vi "Main5states.vi"() -> ()   [LabVIEW 2021]
uses:
  controls/SynchroCheckCentral.ctl
  controls/SynchroCheckCentral_Info.ctl
  controls/SynchroCheckCentral_Data.ctl
  controls/3ph Phasor.ctl
  controls/Phasor.ctl
  controls/AFE_froming_Central.ctl
  controls/AFE_froming_Central_Info.ctl
  controls/AFE_froming_Central_Data.ctl
  controls/references.ctl
  controls/Connected_OPF.ctl
  controls/Connected_OPF_Info.ctl
  controls/Connected_OPF_Data.ctl
  controls/PVemulator_Central.ctl
  controls/PVemulator_Central_Info.ctl
  controls/PVemulator_Central_Data.ctl
  controls/measurements.ctl
  controls/measurements_SC.ctl
  controls/SC_references.ctl
  controls/MeteoBoxCentral.ctl
  controls/MeteoBoxCentral_Info.ctl
  controls/MeteoBoxCentral_Data.ctl
  controls/Setpoints_CDA.ctl
  controls/Setpoints_CDA_ZENONE.ctl
  controls/SCADA_to_SM.ctl
  controls/SCADAOGCentral_Info.ctl
  controls/SCADA_to_SM_Data.ctl
  controls/State Machine.ctl
  <vilib>/Platform/TimedLoop/XDataNode/timing_clust.ctl
  <vilib>/Platform/TimedLoop/XDataNode/nitl_modes.ctl
  <vilib>/Platform/TimedLoop/XDataNode/wakeup.ctl
  controls/PV_facade_central.ctl
  controls/PV_facade_cental_Info.ctl
  controls/PV_facade_central_Data.ctl
  controls/state_2.ctl
  <vilib>/Analysis/baseanly.llb/Mean (DBL).vi
  <vilib>/JDP Science/JSONtext/Next JSON Value.vi
  <vilib>/JDP Science/JSONtext/String Subset.vi
  <vilib>/JDP Science/JSONtext/Parsing/Advance past next JSON Value (inlined COPY).vi
  <vilib>/JDP Science/JSONtext/Parsing/Advance past whitespace.vi
  <vilib>/JDP Science/JSONtext/Parsing/Advance past String.vi
  <vilib>/JDP Science/JSONtext/Parsing/Advance past Number.vi
  <vilib>/JDP Science/JSONtext/Parsing/Advance past Line Ending.vi
  <vilib>/JDP Science/JSONtext/Parsing/Parse Full Path or Item Name.vi
  <vilib>/JDP Science/JSONtext/Parsing/Advance past Array.vi
  <vilib>/JDP Science/JSONtext/Parsing/Advance past Object.vi
  <vilib>/JDP Science/JSONtext/support/Error Cluster From Code.vi
  <vilib>/JDP Science/JSONtext/Offset/Find Item Locations by Path.vi
  <vilib>/Utility/file.llb/Read Delimited Spreadsheet (DBL).vi
  <vilib>/Platform/TimedLoop/TimeConversion.llb/rt-milliseconds-to-rel-time.vi
  <vilib>/Platform/TimedLoop/XDataNode/XDataNode.xnode
  <vilib>/Platform/TimedLoop/XDataNode/XDNodeRunTimeDep.lvlib
  <vilib>/JDP Science/JSONtext/JSONtext.lvlib
  <userlib>/_OpenG.lib/boolean/boolean.llb/openg_boolean__ogtk.lvlib
  <vilib>/ptbypt/NI_PtbyPt.lvlib
  <vilib>/Analysis/NI_AALBase.lvlib
panel:
  in  "IN cOPF 2":T1={"Info"={"Resource"="Zenone", "Problem"=0.0, "Timestamp"=0.0}, "Data"={"Operation_mode"="Grid connected", "solution_feasible"=0.0, "Optimal_slack"="AFE 1", "setpoints"=[], "upper_layer_grid_info"={"Frequency"=0.0, "Angle"=0.0, "Magnitude"=0.0}, "SC_soc"=0.0, "PV"={"perun"=0.0, "solarmax"=0.0, "facade"=0.0, "emul4"=0.0, "emul5"=0.0, "emul6"=0.0, "emul7"=0.0}, "P_pv_facade"=0.0}}
  out "OUT cOPF 2":T1={"Info"={"Resource"="Zenone", "Problem"=0.0, "Timestamp"=0.0}, "Data"={"Operation_mode"="Grid connected", "solution_feasible"=0.0, "Optimal_slack"="AFE 1", "setpoints"=[], "upper_layer_grid_info"={"Frequency"=0.0, "Angle"=0.0, "Magnitude"=0.0}, "SC_soc"=0.0, "PV"={"perun"=0.0, "solarmax"=0.0, "facade"=0.0, "emul4"=0.0, "emul5"=0.0, "emul6"=0.0, "emul7"=0.0}, "P_pv_facade"=0.0}}
  in  "Stop 2":bool
  out "Iteration Duration":dbl
  out "old_sp_island_bool":bool=TRUE
  out "old_sp_island":dbl[](array[numeric])
  out "V_freq_for_island":dbl
  out "V_freq":dbl
  out "V angle":cluster{"output":dbl}(graph)
  in  "Reset_angle":bool
  in  "SampleSize 2":u8=33
  out "SOC":cluster{"mean":dbl}(graph)
  out "V_control_fix_for_island":dbl
  out "V control":cluster{"output":dbl}(graph)
  out "V_control":dbl
  out "V_afe":dbl
  out "V_upstream":dbl
  in  "Reset_magnitude":bool
  out "SCADA data":bool
  in  "SCADA":T4={"Info"={"Resource"="MeteoBox", "Problem"=FALSE, "Timestamp"=0.0}, "Data"={"Voltage mag"=[], "Voltage angle"=[]}}
  in  "to connected-island":bool
  in  "OUT":T7
  in  "Real_SOC":bool
  out "time connected":timestamp
  out "time island":timestamp
  out "P_bess_island":dbl
  out "P_bess_connected":dbl
  out "P_pv_facade":dbl
  in  "SOC":dbl=40.0
  in  "IN Meteo":T9={"Info"={"Resource"="MeteoBox", "Problem"=FALSE, "Timestamp"=0.0}, "Data"={"GI"=0.0, "GHI"=0.0, "GVI"=0.0, "Tair"=0.0, "Tcell roof"=0.0, "Global_Total_Irr"=0.0, "Diffused_Irr"=0.0, "Tcell facade"=0.0, "PV_mpp"={"perun"=0.0, "solarmax"=0.0, "facade"=0.0, "emul4"=0.0, "emul5"=0.0, "emul6"=0.0, "emul7"=0.0}}}
  out "SC_soc":dbl
  out "delta angle":dbl
  in  "Send sp DC?":bool
  in  "Send sp AC?":bool
  out "Zenone_Q":dbl
  out "Zenone_P":dbl
  out "forming SC?":bool
  out "OUT PV+SC":T12={"Info"={"Resource"="Zenone", "Problem"=FALSE, "Timestamp"=0.0}, "Data"={"Status 1"=FALSE, "Status 2"=FALSE, "measurements"={"V_PV1"=0.0, "V_CAP1"=0.0, "V_PV2"=0.0, "V_CAP2"=0.0, "V_grid2"=0.0, "V_PV3"=0.0, "V_CAP3"=0.0, "V_grid3"=0.0, "V_PV4"=0.0, "V_CAP4"=0.0, "V_grid4"=0.0, "V_grid1"=0.0, "P1"=0.0, "P2"=0.0, "P3"=0.0, "P4"=0.0}, "Status 3"=FALSE, "Status 4"=FALSE, "measurements SC"={"V_SC"=0.0, "V_CAP"=0.0, "V_grid"=0.0, "P"=0.0, "SOC"=0.0}, "Status SC"=FALSE, "Forming/Following"=FALSE, "Start forming"=FALSE, "SC references"={"Vdc"=0.0, "Pdc"=0.0}, "Start following"=FALSE}}
  out "PV data":bool
  out "AFE data":bool
  out "synchro data":bool
  in  "IN PV+SC":T12={"Info"={"Resource"="Zenone", "Problem"=FALSE, "Timestamp"=0.0}, "Data"={"Status 1"=FALSE, "Status 2"=FALSE, "measurements"={"V_PV1"=0.0, "V_CAP1"=0.0, "V_PV2"=0.0, "V_CAP2"=0.0, "V_grid2"=0.0, "V_PV3"=0.0, "V_CAP3"=0.0, "V_grid3"=0.0, "V_PV4"=0.0, "V_CAP4"=0.0, "V_grid4"=0.0, "V_grid1"=0.0, "P1"=0.0, "P2"=0.0, "P3"=0.0, "P4"=0.0}, "Status 3"=FALSE, "Status 4"=FALSE, "measurements SC"={"V_SC"=0.0, "V_CAP"=0.0, "V_grid"=0.0, "P"=0.0, "SOC"=0.0}, "Status SC"=FALSE, "Forming/Following"=FALSE, "Start forming"=FALSE, "SC references"={"Vdc"=0.0, "Pdc"=0.0}, "Start following"=FALSE}}
  out "iOPF data":bool
  out "cOPF data":bool
  in  "IN AFE":T18={"Info"={"Resource"="Zenone", "Problem"=FALSE, "Timestamp"=0.0}, "Data"={"Start forming 1"=FALSE, "Forming/Following"=[], "Start forming 2"=FALSE, "measurements"={"Vdc1"=0.0, "P1"=0.0, "Vdc2"=0.0, "P2"=0.0, "Q2"=0.0, "Vdc3"=0.0, "P3"=0.0, "Q3"=0.0, "Vdc4"=0.0, "P4"=0.0, "Q4"=0.0, "Q1"=0.0}, "Status"=[], "references"={"Vdc1"=0.0, "Vdc2"=0.0, "Qac2"=0.0, "Vdc3"=0.0, "Qac3"=0.0, "Vdc4"=0.0, "Qac4"=0.0, "Qac1"=0.0, "V_arg2"=0.0, "V_abs2"=0.0, "V_abs1"=0.0, "V_arg1"=0.0, "freq1"=0.0, "freq2"=0.0}, "Start following 1"=FALSE, "Start following 2"=FALSE}}
  in  "IN cOPF":T1={"Info"={"Resource"="Zenone", "Problem"=0.0, "Timestamp"=0.0}, "Data"={"Operation_mode"="Grid connected", "solution_feasible"=0.0, "Optimal_slack"="AFE 1", "setpoints"=[], "upper_layer_grid_info"={"Frequency"=0.0, "Angle"=0.0, "Magnitude"=0.0}, "SC_soc"=0.0, "PV"={"perun"=0.0, "solarmax"=0.0, "facade"=0.0, "emul4"=0.0, "emul5"=0.0, "emul6"=0.0, "emul7"=0.0}, "P_pv_facade"=0.0}}
  in  "IN iOPF":T1={"Info"={"Resource"="Zenone", "Problem"=0.0, "Timestamp"=0.0}, "Data"={"Operation_mode"="Grid connected", "solution_feasible"=0.0, "Optimal_slack"="AFE 1", "setpoints"=[], "upper_layer_grid_info"={"Frequency"=0.0, "Angle"=0.0, "Magnitude"=0.0}, "SC_soc"=0.0, "PV"={"perun"=0.0, "solarmax"=0.0, "facade"=0.0, "emul4"=0.0, "emul5"=0.0, "emul6"=0.0, "emul7"=0.0}, "P_pv_facade"=0.0}}
  in  "IN synchro":T22={"Info"={"Resource"="SyncroCheck", "Problem"=FALSE, "Timestamp"=0.0}, "Data"={"close/open relay"=TRUE, "Operation mode"="Grid connected", "V_Downstream"={"Phase A"={"Frequency"=0.0, "Magnitude"=0.0, "Angle [Deg]"=0.0}, "Phase B"={"Frequency"=0.0, "Magnitude"=0.0, "Angle [Deg]"=0.0}, "Phase C"={"Frequency"=0.0, "Magnitude"=0.0, "Angle [Deg]"=0.0}, "Phase N"={"Frequency"=0.0, "Magnitude"=0.0, "Angle [Deg]"=0.0}}, "V_UpStream"={"Phase A"={"Frequency"=0.0, "Magnitude"=0.0, "Angle [Deg]"=0.0}, "Phase B"={"Frequency"=0.0, "Magnitude"=0.0, "Angle [Deg]"=0.0}, "Phase C"={"Frequency"=0.0, "Magnitude"=0.0, "Angle [Deg]"=0.0}, "Phase N"={"Frequency"=0.0, "Magnitude"=0.0, "Angle [Deg]"=0.0}}, "Synchronised?"=TRUE}}
  out "OUT iOPF":T1={"Info"={"Resource"="Zenone", "Problem"=0.0, "Timestamp"=0.0}, "Data"={"Operation_mode"="Grid connected", "solution_feasible"=0.0, "Optimal_slack"="AFE 1", "setpoints"=[], "upper_layer_grid_info"={"Frequency"=0.0, "Angle"=0.0, "Magnitude"=0.0}, "SC_soc"=0.0, "PV"={"perun"=0.0, "solarmax"=0.0, "facade"=0.0, "emul4"=0.0, "emul5"=0.0, "emul6"=0.0, "emul7"=0.0}, "P_pv_facade"=0.0}}
  out "OUT cOPF":T1={"Info"={"Resource"="Zenone", "Problem"=0.0, "Timestamp"=0.0}, "Data"={"Operation_mode"="Grid connected", "solution_feasible"=0.0, "Optimal_slack"="AFE 1", "setpoints"=[], "upper_layer_grid_info"={"Frequency"=0.0, "Angle"=0.0, "Magnitude"=0.0}, "SC_soc"=0.0, "PV"={"perun"=0.0, "solarmax"=0.0, "facade"=0.0, "emul4"=0.0, "emul5"=0.0, "emul6"=0.0, "emul7"=0.0}, "P_pv_facade"=0.0}}
  out "OUT AFE":T18={"Info"={"Resource"="Zenone", "Problem"=FALSE, "Timestamp"=0.0}, "Data"={"Start forming 1"=FALSE, "Forming/Following"=[], "Start forming 2"=FALSE, "measurements"={"Vdc1"=0.0, "P1"=0.0, "Vdc2"=0.0, "P2"=0.0, "Q2"=0.0, "Vdc3"=0.0, "P3"=0.0, "Q3"=0.0, "Vdc4"=0.0, "P4"=0.0, "Q4"=0.0, "Q1"=0.0}, "Status"=[], "references"={"Vdc1"=0.0, "Vdc2"=0.0, "Qac2"=0.0, "Vdc3"=0.0, "Qac3"=0.0, "Vdc4"=0.0, "Qac4"=0.0, "Qac1"=0.0, "V_arg2"=0.0, "V_abs2"=0.0, "V_abs1"=0.0, "V_arg1"=0.0, "freq1"=0.0, "freq2"=0.0}, "Start following 1"=FALSE, "Start following 2"=FALSE}}
  out "OUT Synchro":T22={"Info"={"Resource"="SyncroCheck", "Problem"=FALSE, "Timestamp"=0.0}, "Data"={"close/open relay"=TRUE, "Operation mode"="Grid connected", "V_Downstream"={"Phase A"={"Frequency"=0.0, "Magnitude"=0.0, "Angle [Deg]"=0.0}, "Phase B"={"Frequency"=0.0, "Magnitude"=0.0, "Angle [Deg]"=0.0}, "Phase C"={"Frequency"=0.0, "Magnitude"=0.0, "Angle [Deg]"=0.0}, "Phase N"={"Frequency"=0.0, "Magnitude"=0.0, "Angle [Deg]"=0.0}}, "V_UpStream"={"Phase A"={"Frequency"=0.0, "Magnitude"=0.0, "Angle [Deg]"=0.0}, "Phase B"={"Frequency"=0.0, "Magnitude"=0.0, "Angle [Deg]"=0.0}, "Phase C"={"Frequency"=0.0, "Magnitude"=0.0, "Angle [Deg]"=0.0}, "Phase N"={"Frequency"=0.0, "Magnitude"=0.0, "Angle [Deg]"=0.0}}, "Synchronised?"=TRUE}}
  out "setpoints":dbl[](array[numeric])
  in  "nb instances":i16=7
  out "optimal_slack":string(combo)="AFE 1"
  out "iOPF valid":bool
  out "forming AFE?":bool
  out "cOPF valid?":bool
  out "synchronised?":bool
  in  "to grid connection":bool
  in  "to prepare for grid connection":bool
  in  "to island":bool
  in  "Stop":bool
  in  "to prepare for island":bool
  # "32.58"
  # "Islanding Manoeuvre - State Machine"
  # "synchronised"
  # "opf connected OK"
  # "opf island OK"
  # "forming AFE?"
  # "forming SC?"
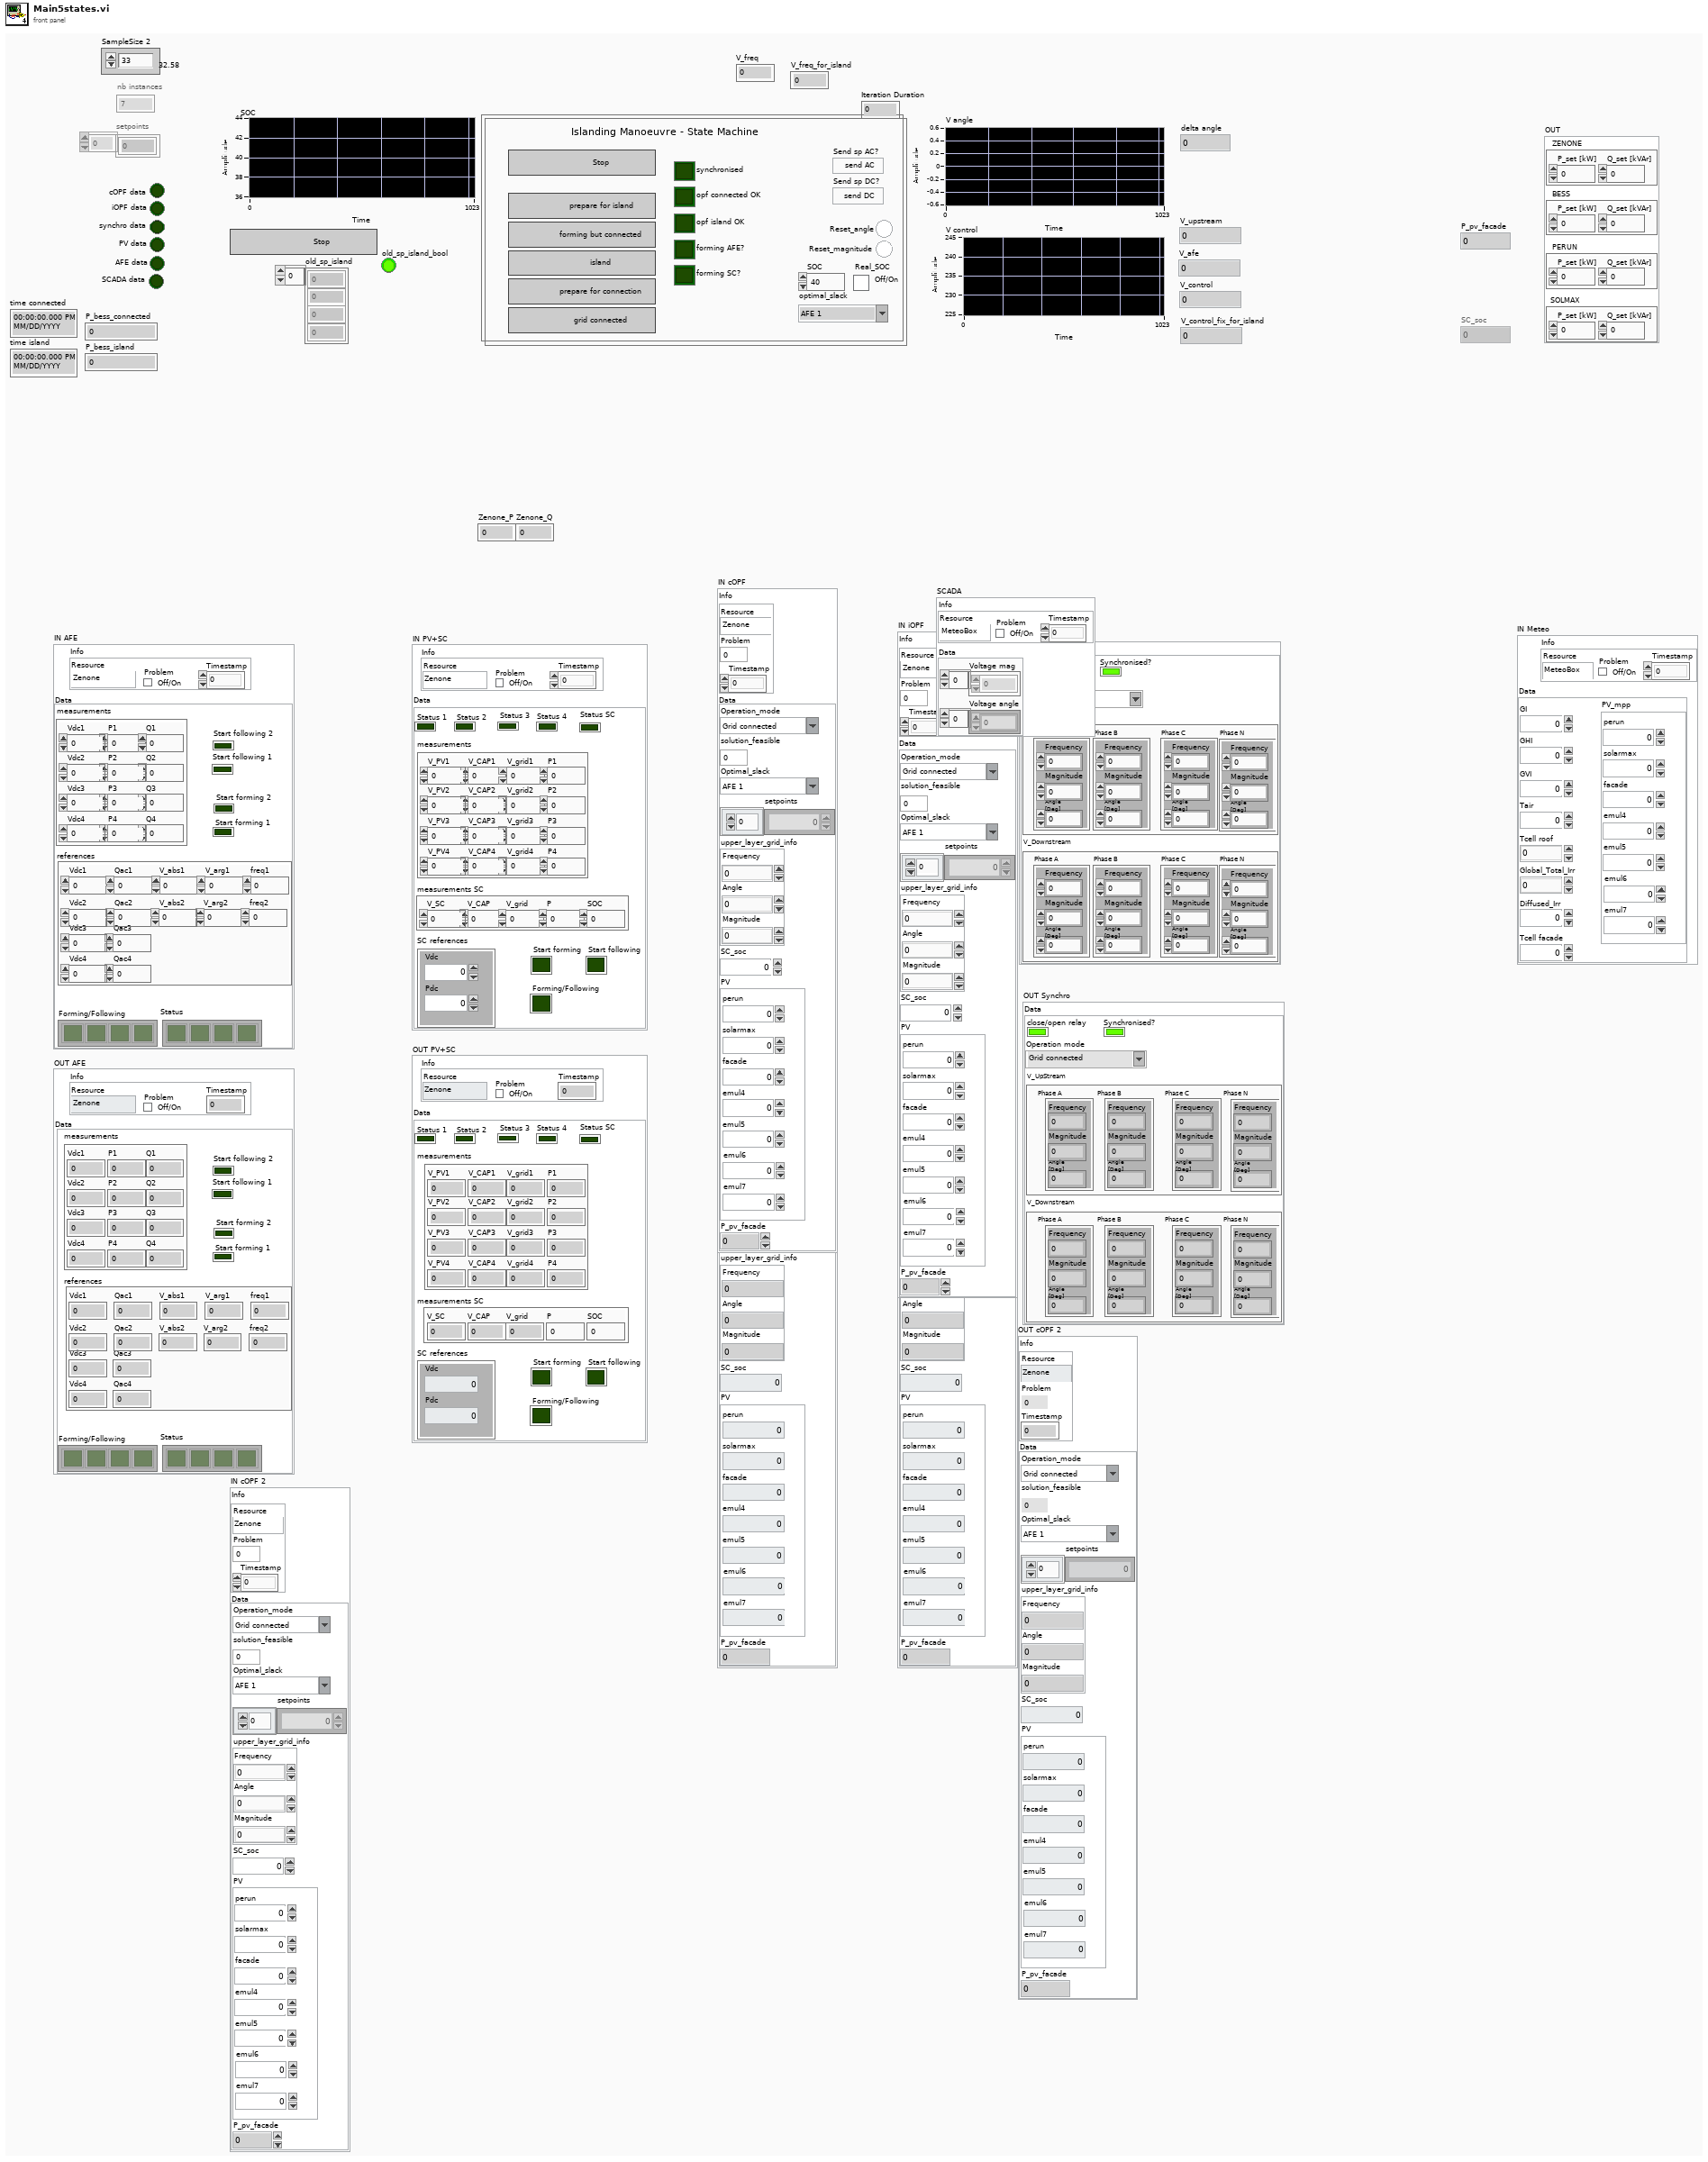
[diagram p1: front panel]
types:
  T1 = typedef "Connected_OPF.ctl" = cluster{"Info":T2, "Data":T3}
  T2 = typedef "Connected_OPF_Info.ctl" = cluster{"Resource":string, "Problem":dbl, "Timestamp":dbl}
  T3 = typedef "Connected_OPF_Data.ctl" = cluster{"Operation_mode":string, "solution_feasible":dbl, "Optimal_slack":string, "setpoints":dbl[], "upper_layer_grid_info":cluster{"Frequency":dbl, "Angle":dbl, "Magnitude":dbl}, "SC_soc":dbl, "PV":cluster{"perun":dbl, "solarmax":dbl, "facade":dbl, "emul4":dbl, "emul5":dbl, "emul6":dbl, "emul7":dbl}, "P_pv_facade":dbl}
  T4 = typedef "SCADA_to_SM.ctl" = cluster{"Info":T5, "Data":T6}
  T5 = typedef "SCADAOGCentral_Info.ctl" = cluster{"Resource":string, "Problem":bool, "Timestamp":dbl}
  T6 = typedef "SCADA_to_SM_Data.ctl" = cluster{"Voltage mag":dbl[], "Voltage angle":dbl[]}
  T7 = typedef "Setpoints_CDA.ctl" = cluster{"ZENONE":T8, "BESS":T8, "PERUN":T8, "SOLMAX":T8}
  T8 = typedef "Setpoints_CDA_ZENONE.ctl" = cluster{"P_set [kW]":dbl, "Q_set [kVAr]":dbl}
  T9 = typedef "MeteoBoxCentral.ctl" = cluster{"Info":T10, "Data":T11}
  T10 = typedef "MeteoBoxCentral_Info.ctl" = cluster{"Resource":string, "Problem":bool, "Timestamp":dbl}
  T11 = typedef "MeteoBoxCentral_Data.ctl" = cluster{"GI":dbl, "GHI":dbl, "GVI":dbl, "Tair":dbl, "Tcell roof":dbl, "Global_Total_Irr":dbl, "Diffused_Irr":dbl, "Tcell facade":dbl, "PV_mpp":cluster{"perun":dbl, "solarmax":dbl, "facade":dbl, "emul4":dbl, "emul5":dbl, "emul6":dbl, "emul7":dbl}}
  T12 = typedef "PVemulator_Central.ctl" = cluster{"Info":T13, "Data":T14}
  T13 = typedef "PVemulator_Central_Info.ctl" = cluster{"Resource":string, "Problem":bool, "Timestamp":dbl}
  T14 = typedef "PVemulator_Central_Data.ctl" = cluster{"Status 1":bool, "Status 2":bool, "measurements":T15, "Status 3":bool, "Status 4":bool, "measurements SC":T16, "Status SC":bool, "Forming/Following":bool, "Start forming":bool, "SC references":T17, "Start following":bool}
  T15 = typedef "measurements.ctl" = cluster{"V_PV1":dbl, "V_CAP1":dbl, "V_PV2":dbl, "V_CAP2":dbl, "V_grid2":dbl, "V_PV3":dbl, "V_CAP3":dbl, "V_grid3":dbl, "V_PV4":dbl, "V_CAP4":dbl, "V_grid4":dbl, "V_grid1":dbl, "P1":dbl, "P2":dbl, "P3":dbl, "P4":dbl}
  T16 = typedef "measurements_SC.ctl" = cluster{"V_SC":dbl, "V_CAP":dbl, "V_grid":dbl, "P":dbl, "SOC":dbl}
  T17 = typedef "SC_references.ctl" = cluster{"Vdc":dbl, "Pdc":dbl}
  T18 = typedef "AFE_froming_Central.ctl" = cluster{"Info":T19, "Data":T20}
  T19 = typedef "AFE_froming_Central_Info.ctl" = cluster{"Resource":string, "Problem":bool, "Timestamp":dbl}
  T20 = typedef "AFE_froming_Central_Data.ctl" = cluster{"Start forming 1":bool, "Forming/Following":bool[], "Start forming 2":bool, "measurements":cluster{"Vdc1":dbl, "P1":dbl, "Vdc2":dbl, "P2":dbl, "Q2":dbl, "Vdc3":dbl, "P3":dbl, "Q3":dbl, "Vdc4":dbl, "P4":dbl, "Q4":dbl, "Q1":dbl}, "Status":bool[], "references":T21, "Start following 1":bool, "Start following 2":bool}
  T21 = typedef "references.ctl" = cluster{"Vdc1":dbl, "Vdc2":dbl, "Qac2":dbl, "Vdc3":dbl, "Qac3":dbl, "Vdc4":dbl, "Qac4":dbl, "Qac1":dbl, "V_arg2":dbl, "V_abs2":dbl, "V_abs1":dbl, "V_arg1":dbl, "freq1":dbl, "freq2":dbl}
  T22 = typedef "SynchroCheckCentral.ctl" = cluster{"Info":T23, "Data":T24}
  T23 = typedef "SynchroCheckCentral_Info.ctl" = cluster{"Resource":string, "Problem":bool, "Timestamp":dbl}
  T24 = typedef "SynchroCheckCentral_Data.ctl" = cluster{"close/open relay":bool, "Operation mode":string, "V_Downstream":T25, "V_UpStream":T25, "Synchronised?":bool}
  T25 = typedef "3ph Phasor.ctl" = cluster{"Phase A":T26, "Phase B":T26, "Phase C":T26, "Phase N":T26}
  T26 = typedef "Phasor.ctl" = cluster{"Frequency":dbl, "Magnitude":dbl, "Angle [Deg]":dbl}
  T27 = typedef "State Machine.ctl" = enum16{"Grid connected", "Prepare for island", "Forming but connected", "Island", "Prepare for connection"}
  T28 = typedef "XDNodeRunTimeDep.lvlib/timing_clust.ctl" = cluster{"Expected End [f-1]":u64, "Actual End [f-1]":u64, "Finished Late? [f-1]":bool, "Expected End [i-1]":u64, "Actual End [i-1]":u64, "Finished Late? [i-1]":bool, "Expected Start [i]":u64, "Actual Start [i]":u64, "Expected Start [f]":u64, "Actual Start [f]":u64, "Source Name":string, "Structure Name":string, "Period":i64, "Deadline":i64, "Offset":i64, "Start":i64, "Priority":i32, "Timeout":i32, "Mode":T29, "Wakeup Reason":T30, "Error":errorcluster, "Source Type":string, "Secondary Source Type":string, "Global End Time":u64, "Global Start Time":u64, "Frame Duration":u64, "Iteration Duration":u64, "Assigned CPU":i32, "I/O Scan Engine Mode":u32}
  T29 = typedef "XDNodeRunTimeDep.lvlib/nitl_modes.ctl" = enum32{"No Change", "Process missed periods, maintain original phase", "Discard missed periods, maintain original phase", "Process missed periods, ignore original phase", "Discard missed periods, ignore original phase"}
  T30 = typedef "XDNodeRunTimeDep.lvlib/wakeup.ctl" = enum32{"Normal", "Aborted", "Asynchronous wakeup", "Timing source error", "Timed loop error", "Timeout"}
  T31 = typedef "PV_facade_central.ctl" = cluster{"Info":T32, "Data":T33}
  T32 = typedef "PV_facade_cental_Info.ctl" = cluster{"Resource":string, "Problem":bool, "Timestamp":dbl}
  T33 = typedef "PV_facade_central_Data.ctl" = cluster{"P":dbl, "Q":dbl, "Pset":dbl, "Qset":dbl}
  T34 = typedef "state_2.ctl" = string
  T35 = cluster{"Frequency":dbl, "Angle":dbl, "Magnitude":dbl}
  T36 = cluster{"perun":dbl, "solarmax":dbl, "facade":dbl, "emul4":dbl, "emul5":dbl, "emul6":dbl, "emul7":dbl}
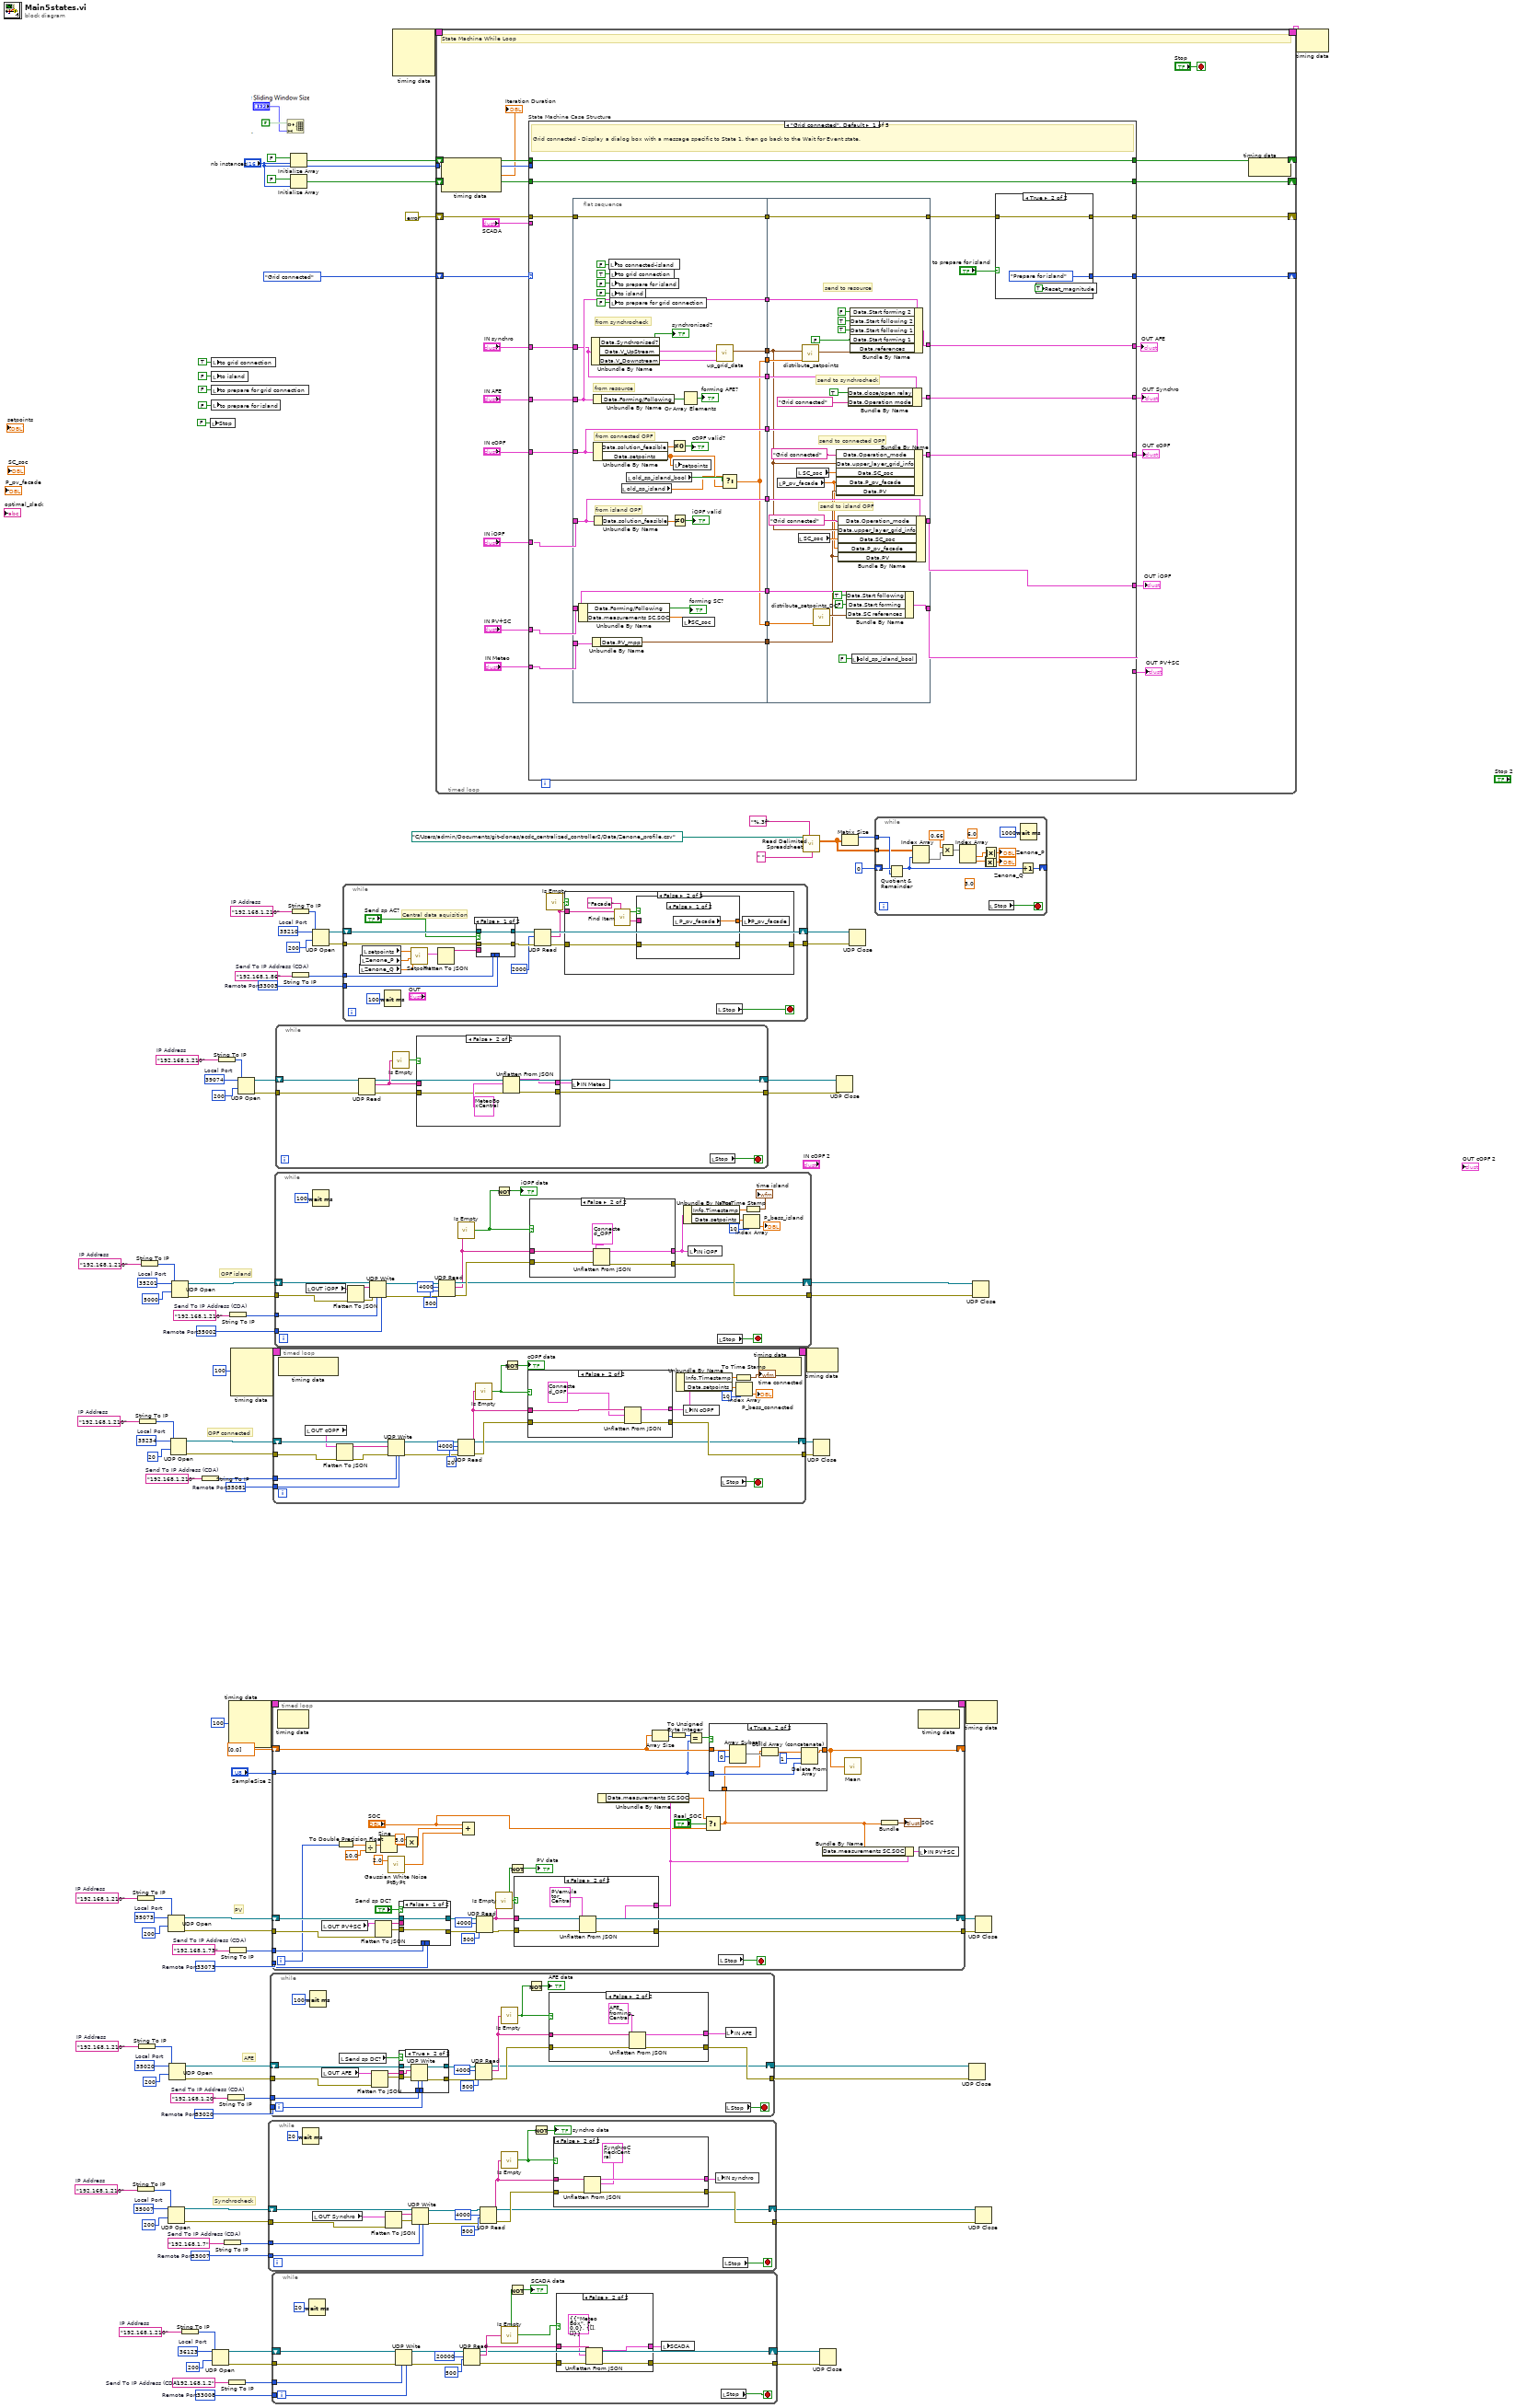
[diagram p0: block diagram]
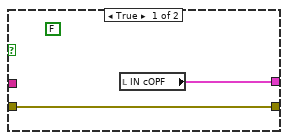
[diagram p2: hidden frame]
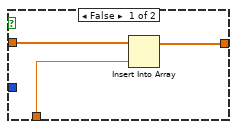
[diagram p3: hidden frame]
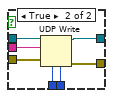
[diagram p4: hidden frame]
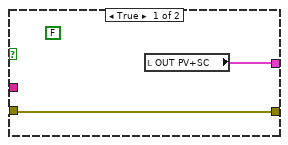
[diagram p5: hidden frame]
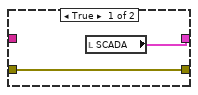
[diagram p6: hidden frame]
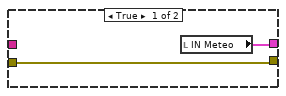
[diagram p7: hidden frame]
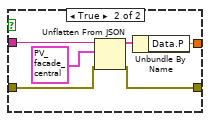
[diagram p9: hidden frame]
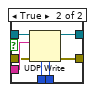
[diagram p10: hidden frame]
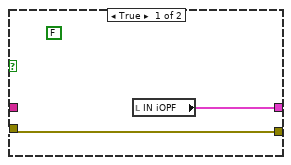
[diagram p11: hidden frame]
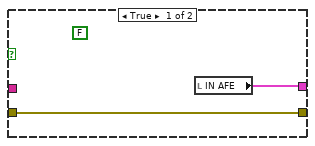
[diagram p13: hidden frame]
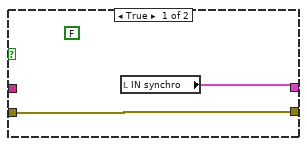
[diagram p14: hidden frame]
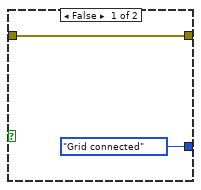
[diagram p15: hidden frame]
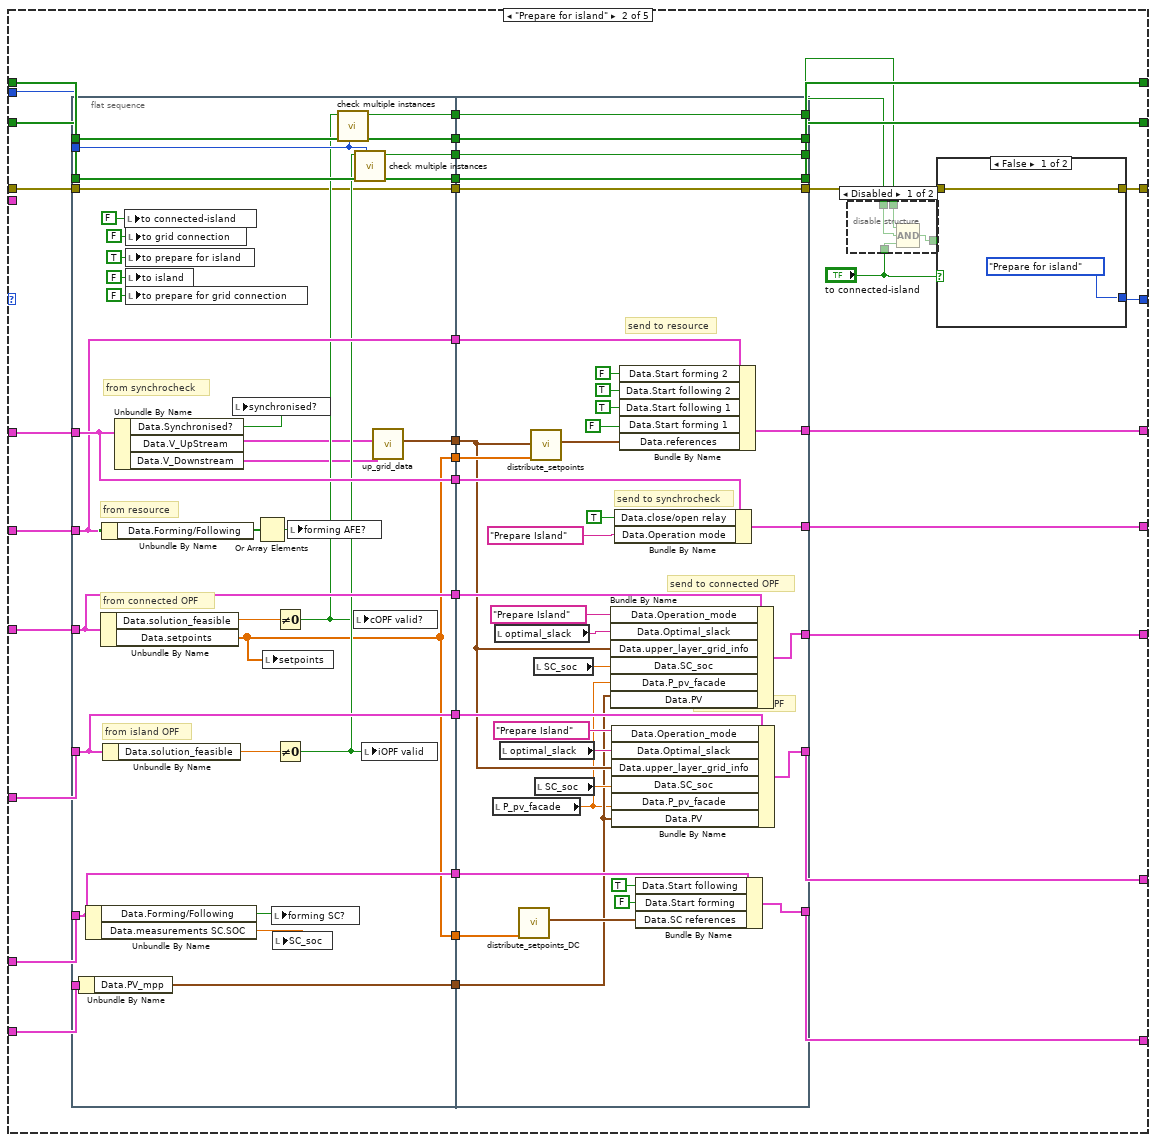
[diagram p16: hidden frame]
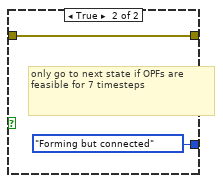
[diagram p18: hidden frame]
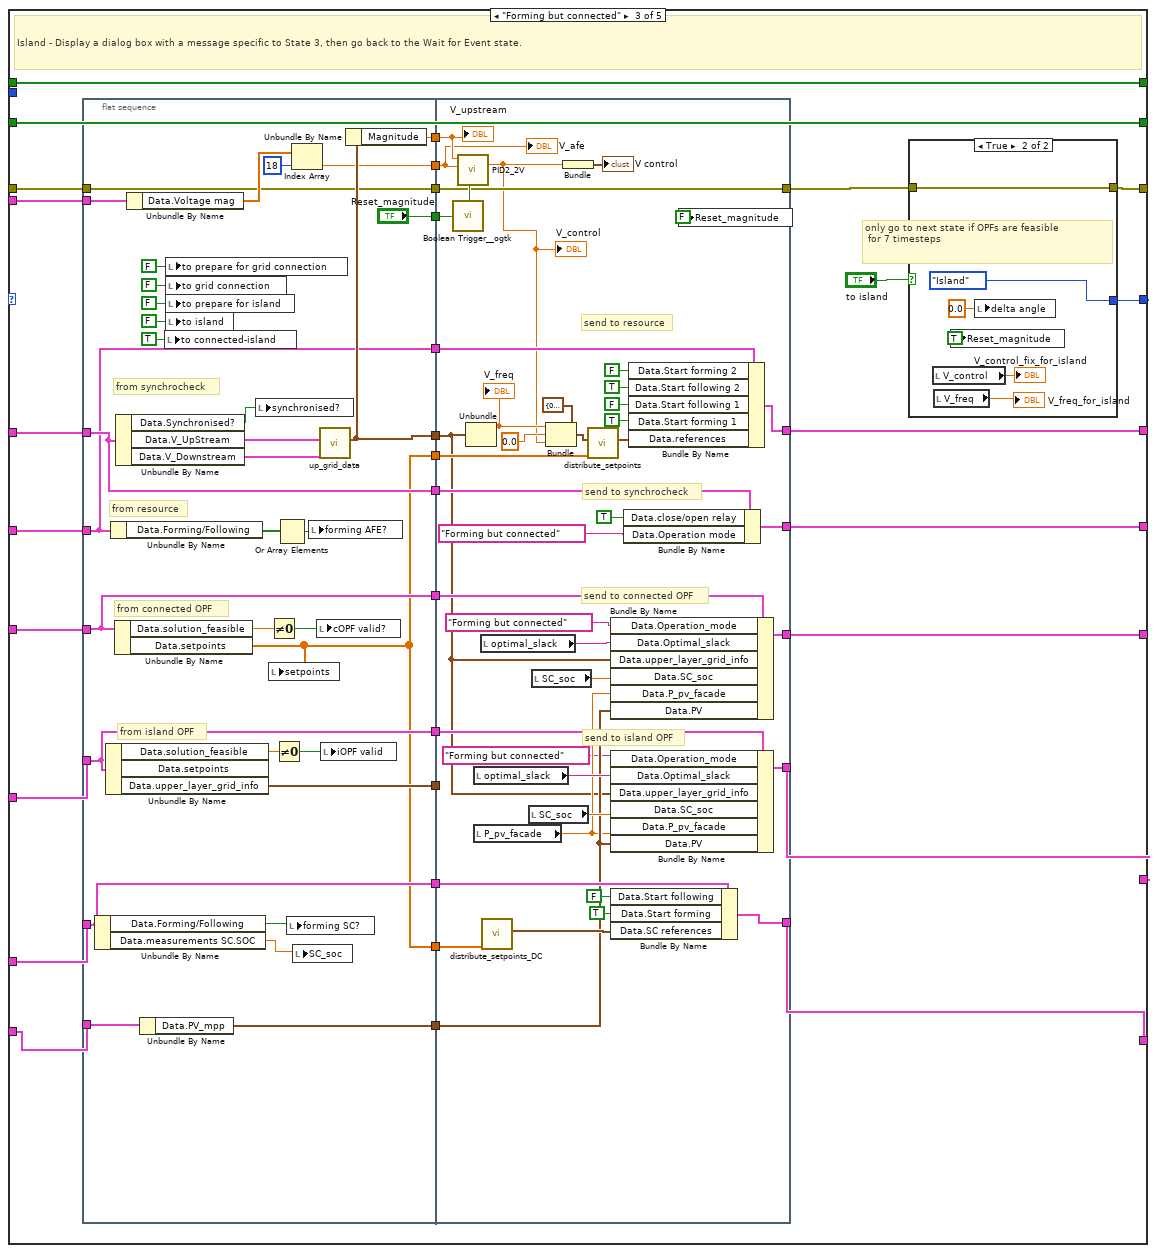
[diagram p19: hidden frame]
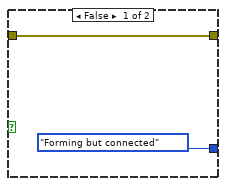
[diagram p20: hidden frame]
diagram:
  w1 = u16 35081  # Remote Port
  w3 = "192.168.1.210"  # Send To IP Address (CDA)
  w15 = u16 33008  # Remote Port
  w19 = "192.168.1.2"  # Send To IP Address (CDA)
  w20 = u16 36123  # Local Port
  w22 = "192.168.1.210"  # IP Address
  w29 = u16 39074  # Local Port
  w31 = "192.168.1.210"  # IP Address
  w40 = u16 33003  # Remote Port
  w42 = "192.168.1.86"  # Send To IP Address (CDA)
  w44 = u16 35210  # Local Port
  w46 = "192.168.1.210"  # IP Address
  w68 = u16 33073  # Remote Port
  w69 = "192.168.1.73"  # Send To IP Address (CDA)
  w64 = u16 33020  # Remote Port
  w72 = "192.168.1.20"  # Send To IP Address (CDA)
  w59 = u16 33007  # Remote Port
  w73 = "192.168.1.7"  # Send To IP Address (CDA)
  w74 = u16 35007  # Local Port
  w76 = "192.168.1.210"  # IP Address
  w78 = u16 35020  # Local Port
  w80 = "192.168.1.210"  # IP Address
  w82 = u16 35073  # Local Port
  w84 = "192.168.1.210"  # IP Address
  w87 = u16 35002  # Remote Port
  w88 = "192.168.1.210"  # Send To IP Address (CDA)
  w95 = u16 35234  # Local Port
  w97 = "192.168.1.210"  # IP Address
  w101 = u16 35201  # Local Port
  w103 = "192.168.1.210"  # IP Address
  # "Synchrocheck"
  # "AFE"
  # "PV"
  # "OPF connected"
  # "OPF island"
  n1 = String To IP(1:w76) -> (0:w77:u32)
  n2 = String To IP(1:w84) -> (0:w85:u32)
  n3 = String To IP(1:w80) -> (0:w81:u32)
  n4 = String To IP(1:w97) -> (0:w98:u32)
  n5 = String To IP(1:w103) -> (0:w104:u32)
  n6 = UDP Open(7:w77, 9:200 ("timeout ms (25000)"), 11:w74) -> (port=w62:refnum<k16>, 0:w61:errorcluster)  [unwired: 2 in, 1 out]
  n7 = UDP Open(7:w85, 9:200 ("timeout ms (25000)"), 11:w82) -> (port=w71:refnum<k16>, 0:w70:errorcluster)  [unwired: 2 in, 1 out]
  n8 = UDP Open(7:w81, 9:200 ("timeout ms (25000)"), 11:w78) -> (port=w66:refnum<k16>, 0:w65:errorcluster)  [unwired: 2 in, 1 out]
  n9 = UDP Open(7:w98, 9:20 ("timeout ms (25000)"), 11:w95) -> (port=w94:refnum<k16>, 0:w93:errorcluster)  [unwired: 2 in, 1 out]
  n10 = UDP Open(7:w104, 9:5000 ("timeout ms (25000)"), 11:w101) -> (port=w100:refnum<k16>, 0:w99:errorcluster)  [unwired: 2 in, 1 out]
  n11 = String To IP(1:w22) -> (0:w23:u32)
  n12 = String To IP(1:w3) -> (0:w2:u32)
  n13 = local write "Stop"(FALSE ("Stop")) -> ()
  n14 = local write "to grid connection"(TRUE ("to grid connection")) -> ()
  n15 = local write "to island"(FALSE ("to island")) -> ()
  n16 = local write "to prepare for grid connection"(FALSE ("to prepare for grid connection")) -> ()
  n17 = local write "to prepare for island"(FALSE ("to prepare for island")) -> ()
  n18 = UDP Open(7:w23, 9:200 ("timeout ms (25000)"), 11:w20) -> (port=w18:refnum<k16>, 0:w17:errorcluster)  [unwired: 2 in, 1 out]
  n19 = String To IP(1:w31) -> (0:w32:u32)
  n20 = String To IP(1:w73) -> (0:w60:u32)
  n21 = String To IP(1:w72) -> (0:w63:u32)
  n22 = node-c288(i64 100 ("Period")) -> (w9:T28)  [unwired: 3 in]
  n23 = String To IP(1:w19) -> (0:w16:u32)
  n24 = String To IP(1:w69) -> (0:w67:u32)
  n25 = String To IP(1:w88) -> (0:w86:u32)
  n26 = node-c288(i64 100 ("Period")) -> (w6:T28)  [unwired: 3 in]
  n27 = UDP Open(7:w32, 9:200 ("timeout ms (25000)"), 11:w29) -> (port=w28:refnum<k16>, 0:w27:errorcluster)  [unwired: 2 in, 1 out]
  n28 = while {
    tunnel: w60 -> [w133]
    tunnel: w59 -> [w132]
    shift-right: [w118] -> w58
    shift-left: w62 -> [w116]
    tunnel: w61 -> [w114]
    tunnel: [w119] -> w57
    stop <- w121 stop-if-true
    n29 = Wait (ms)(milliseconds to wait=u32 20) -> ()  [unwired: 1 out]
    n30 = local read "OUT Synchro"() -> (w126:T22)
    n31 = Flatten To JSON(anything=w126, error in (no error)=w114) -> (JSON string=w120:string, 11:w127:errorcluster)  [unwired: 1 in]
    n32 = UDP Write(address=w133, port or service name=w132, connection ID=w116, data in=w120, 8:w127) -> (error out=w115:errorcluster, 3:w117:refnum<k16>)  [unwired: 1 in]
    n33 = UDP Read(connection ID=w117, max size (548)=4000, timeout ms (25000)=500, 8:w115) -> (data out=w131:string, error out=w123:errorcluster, 3:w118:refnum<k16>)  [unwired: 2 out]
    n34 = call <vilib>:"Is Empty.vi"("JSON"=w131) -> ("Empty"=w124:bool)  [unwired: 4 in]
    n35 = Not(x=w124) -> (.not. x?=→"synchro data":bool)
    n36 = case shown="False" w124 {
      tunnel: w123 -> [w135 w137]
      tunnel: [w134 w140] -> w128
      tunnel: w131 -> [_ w136]
      tunnel: [w135 w139] -> w119
      frame True {
        (unwired) FALSE ("Found")
        n37 = local read "IN synchro"() -> (w134:T22)
      }
      frame False {
        n38 = Unflatten From JSON(JSON string=w136, type and defaults=T22 {"Info"={"Resource"="SyncroCheck", "Problem"=FALSE, "Timestamp"=0.0}, "Data"={"close/open relay"=TRUE, "Operation mode"="Grid connected", "V_Downstream"={"Phase A"={"Frequency"=0.0, "Magnitude"=0.0, "Angle [Deg]"=0.0}, "Phase B"={"Frequency"=0.0, "Magnitude"=0.0, "Angle [Deg]"=0.0}, "Phase C"={"Frequency"=0.0, "Magnitude"=0.0, "Angle [Deg]"=0.0}, "Phase N"={"Frequency"=0.0, "Magnitude"=0.0, "Angle [Deg]"=0.0}}, "V_UpStream"={"Phase A"={"Frequency"=0.0, "Magnitude"=0.0, "Angle [Deg]"=0.0}, "Phase B"={"Frequency"=0.0, "Magnitude"=0.0, "Angle [Deg]"=0.0}, "Phase C"={"Frequency"=0.0, "Magnitude"=0.0, "Angle [Deg]"=0.0}, "Phase N"={"Frequency"=0.0, "Magnitude"=0.0, "Angle [Deg]"=0.0}}, "Synchronised?"=TRUE}} ("IN synchro"), error in (no error)=w137) -> (value=w140:T22, error out=w139:errorcluster)  [unwired: 4 in]
      }
    }
    n39 = local write "IN synchro"(w128) -> ()
    n40 = local read "Stop"() -> (w121:bool)
  }
  n41 = while {
    tunnel: w64 -> [w161]
    tunnel: w63 -> [w160]
    shift-right: [w144] -> w54
    shift-left: w66 -> [w146]
    tunnel: w65 -> [w148]
    tunnel: [w150] -> w53
    stop <- w152 stop-if-true
    n42 = Wait (ms)(milliseconds to wait=u32 100) -> ()  [unwired: 1 out]
    n43 = local read "OUT AFE"() -> (w143:T18)
    n44 = local read "Send sp DC?"() -> (w141:bool)
    n45 = Flatten To JSON(anything=w143, error in (no error)=w148) -> (JSON string=w151:string, 11:w156:errorcluster)  [unwired: 1 in]
    n46 = case shown="True" w141 {
      tunnel: w161 -> [_ w170]
      tunnel: w160 -> [_ w169]
      tunnel: w156 -> [w162 w168]
      tunnel: w151 -> [_ w167]
      tunnel: [w162 w166] -> w149
      tunnel: [w163 w165] -> w147
      tunnel: w146 -> [w163 w164]
      frame False {
      }
      frame True {
        n47 = UDP Write(address=w169, port or service name=w170, connection ID=w164, data in=w167, 8:w168) -> (error out=w166:errorcluster, 3:w165:refnum<k16>)  [unwired: 1 in]
      }
    }
    n48 = UDP Read(connection ID=w147, max size (548)=4000, timeout ms (25000)=500, 8:w149) -> (data out=w145:string, error out=w157:errorcluster, 3:w144:refnum<k16>)  [unwired: 2 out]
    n49 = call <vilib>:"Is Empty.vi"("JSON"=w145) -> ("Empty"=w154:bool)  [unwired: 4 in]
    n50 = Not(x=w154) -> (.not. x?=→"AFE data":bool)
    n51 = case shown="False" w154 {
      tunnel: w157 -> [w172 w176]
      tunnel: [w171 w174] -> w142
      tunnel: w145 -> [_ w175]
      tunnel: [w172 w177] -> w150
      frame True {
        (unwired) FALSE ("Found")
        n52 = local read "IN AFE"() -> (w171:T18)
      }
      frame False {
        n53 = Unflatten From JSON(JSON string=w175, type and defaults=T18 {"Info"={"Resource"="Zenone", "Problem"=FALSE, "Timestamp"=0.0}, "Data"={"Start forming 1"=FALSE, "Forming/Following"=[], "Start forming 2"=FALSE, "measurements"={"Vdc1"=0.0, "P1"=0.0, "Vdc2"=0.0, "P2"=0.0, "Q2"=0.0, "Vdc3"=0.0, "P3"=0.0, "Q3"=0.0, "Vdc4"=0.0, "P4"=0.0, "Q4"=0.0, "Q1"=0.0}, "Status"=[], "references"={"Vdc1"=0.0, "Vdc2"=0.0, "Qac2"=0.0, "Vdc3"=0.0, "Qac3"=0.0, "Vdc4"=0.0, "Qac4"=0.0, "Qac1"=0.0, "V_arg2"=0.0, "V_abs2"=0.0, "V_abs1"=0.0, "V_arg1"=0.0, "freq1"=0.0, "freq2"=0.0}, "Start following 1"=FALSE, "Start following 2"=FALSE}} ("IN AFE"), error in (no error)=w176) -> (value=w174:T18, error out=w177:errorcluster)  [unwired: 4 in]
      }
    }
    n54 = local write "IN AFE"(w142) -> ()
    n55 = local read "Stop"() -> (w152:bool)
  }
  n56 = timed-loop {
    tunnel: w68 -> [w218]
    tunnel: w67 -> [w201]
    shift-right: [w206] -> w56
    shift-left: w71 -> [w209]
    tunnel: w70 -> [w205]
    tunnel: [w203] -> w55
    shift-right: [w185] -> _
    shift-left: dbl[] [0.0] -> [w187]
    tunnel: "SampleSize 2" -> [w179]
    timing: w9 -> [_]
    timing-out: [_] -> w8
    i -> [w186]
    stop <- w210 stop-if-true
    n57 = node-c288() -> ()  [unwired: 1 in, 1 out]
    n58 = local read "OUT PV+SC"() -> (w202:T12)
    n59 = To Double Precision Float(number=w186) -> (double precision float=w198:dbl)
    n60 = Divide(x=w198, y=10.0) -> (x/y=w197:dbl)
    n61 = Flatten To JSON(anything=w202, error in (no error)=w205) -> (JSON string=w211:string, 11:w214:errorcluster)  [unwired: 1 in]
    n62 = Sine(x=w197) -> (sin(x)=w195:dbl)
    n63 = call <vilib>:"Gaussian White Noise PtByPt.vi"("standard deviation"=2.0) -> ("Gaussian white noise"=w194:dbl)  [unwired: 2 in]
    n64 = case shown="False" "Send sp DC?" {
      tunnel: w218 -> [_ w240]
      tunnel: w201 -> [_ w239]
      tunnel: w214 -> [w232 w238]
      tunnel: w211 -> [_ w237]
      tunnel: w209 -> [w233 w236]
      tunnel: [w233 w235] -> w207
      tunnel: [w232 w234] -> w204
      frame False {
      }
      frame True {
        n65 = UDP Write(address=w239, port or service name=w240, connection ID=w236, data in=w237, 8:w238) -> (error out=w234:errorcluster, 3:w235:refnum<k16>)  [unwired: 1 in]
      }
    }
    n66 = Multiply(x=5.0, y=w195) -> (x*y=w192:dbl)
    n67 = Compound Arithmetic op=ADD("SOC", w192, w194) -> ()  [unwired: 1 out]
    n68 = UDP Read(connection ID=w207, max size (548)=4000, timeout ms (25000)=500, 8:w204) -> (data out=w217:string, error out=w215:errorcluster, 3:w206:refnum<k16>)  [unwired: 2 out]
    n69 = call <vilib>:"Is Empty.vi"("JSON"=w217) -> ("Empty"=w212:bool)  [unwired: 4 in]
    n70 = Not(x=w212) -> (.not. x?=→"PV data":bool)
    n71 = case shown="False" w212 {
      tunnel: w215 -> [w242 w245]
      tunnel: [w241 w247] -> w182
      tunnel: w217 -> [_ w244]
      tunnel: [w242 w246] -> w203
      frame True {
        (unwired) FALSE ("Found")
        n72 = local read "OUT PV+SC"() -> (w241:T12)
      }
      frame False {
        n73 = Unflatten From JSON(JSON string=w244, type and defaults=T12 {"Info"={"Resource"="Zenone", "Problem"=FALSE, "Timestamp"=0.0}, "Data"={"Status 1"=FALSE, "Status 2"=FALSE, "measurements"={"V_PV1"=0.0, "V_CAP1"=0.0, "V_PV2"=0.0, "V_CAP2"=0.0, "V_grid2"=0.0, "V_PV3"=0.0, "V_CAP3"=0.0, "V_grid3"=0.0, "V_PV4"=0.0, "V_CAP4"=0.0, "V_grid4"=0.0, "V_grid1"=0.0, "P1"=0.0, "P2"=0.0, "P3"=0.0, "P4"=0.0}, "Status 3"=FALSE, "Status 4"=FALSE, "measurements SC"={"V_SC"=0.0, "V_CAP"=0.0, "V_grid"=0.0, "P"=0.0, "SOC"=0.0}, "Status SC"=FALSE, "Forming/Following"=FALSE, "Start forming"=FALSE, "SC references"={"Vdc"=0.0, "Pdc"=0.0}, "Start following"=FALSE}} ("PV+SC"), error in (no error)=w245) -> (value=w247:T12, error out=w246:errorcluster)  [unwired: 4 in]
      }
    }
    n74 = Unbundle By Name(w182) -> ("Data.measurements SC.SOC"=w181:dbl)
    n75 = Array Size(array=w187) -> (size(s)=w189:i32)
    n76 = To Unsigned Byte Integer(number=w189) -> (unsigned 8bit integer=w183:u8)
    n77 = Equal?(x=w183, y=w179) -> (x = y?=w188:bool)
    n78 = Select(t=w181, s="Real_SOC", f="SOC") -> (s? t:f=w178:dbl)
    n79 = case shown="True" w188 {
      tunnel: [w223 w227] -> w185
      tunnel: w187 -> [w222 w231]
      tunnel: w179 -> [_ w225]
      tunnel: w178 -> [w221 w224]
      frame False {
        n80 = Insert Into Array(array=w222, new element=w221) -> (w223:dbl[])  [unwired: 1 in]
      }
      frame True {
        n81 = Array Subset(array=w231, index=0) -> (w229:dbl[])  [unwired: 1 in]
        n82 = Build Array (concatenate)(w224, w229) -> (w228:dbl[])
        n83 = Delete From Array(array=w228, length=1, index=w225) -> (array with subset deleted=w227:dbl[])  [unwired: 1 out]
      }
    }
    n84 = local read "Stop"() -> (w210:bool)
    n85 = Bundle By Name(cluster=w182, "Data.measurements SC.SOC"=w178) -> (w184:T12)
    n86 = call-poly <vilib>:"Mean.vi"("X"=w185) -> ()  [unwired: 2 out]
    n87 = Bundle("SOC"=w178) -> (→"SOC":cluster{"SOC":dbl})  [unwired: 1 in]
    n88 = node-c288() -> ()  [unwired: 1 in, 1 out]
    n89 = local write "IN PV+SC"(w184) -> ()
  }
  n90 = while {
    tunnel: w16 -> [w258]
    tunnel: w15 -> [w259]
    shift-right: [w249] -> w14
    shift-left: w18 -> [w257]
    tunnel: w17 -> [w256]
    tunnel: [w250] -> w13
    stop <- w248 stop-if-true
    n91 = Wait (ms)(milliseconds to wait=u32 20) -> ()  [unwired: 1 out]
    n92 = UDP Write(address=w258, port or service name=w259, connection ID=w257, 8:w256) -> (error out=w260:errorcluster, 3:w261:refnum<k16>)  [unwired: 2 in]
    n93 = UDP Read(connection ID=w261, max size (548)=20000, timeout ms (25000)=500, 8:w260) -> (data out=w252:string, error out=w253:errorcluster, 3:w249:refnum<k16>)  [unwired: 2 out]
    n94 = call <vilib>:"Is Empty.vi"("JSON"=w252) -> ("Empty"=w254:bool)  [unwired: 4 in]
    n95 = Not(x=w254) -> (.not. x?=→"SCADA data":bool)
    n96 = case shown="False" w254 {
      tunnel: w253 -> [w265 w271]
      tunnel: w252 -> [_ w270]
      tunnel: [w266 w268] -> w251
      tunnel: [w265 w267] -> w250
      frame True {
        n97 = local read "SCADA"() -> (w266:T4)
      }
      frame False {
        n98 = Unflatten From JSON(JSON string=w270, type and defaults=T4 {"Info"={"Resource"="MeteoBox", "Problem"=FALSE, "Timestamp"=0.0}, "Data"={"Voltage mag"=[], "Voltage angle"=[]}} ("Cluster"), error in (no error)=w271) -> (value=w268:T4, error out=w267:errorcluster)  [unwired: 4 in]
      }
    }
    n99 = local write "SCADA"(w251) -> ()
    n100 = local read "Stop"() -> (w248:bool)
  }
  n101 = timed-loop {
    shift-right: [w284] -> w90
    shift-left: w94 -> [w288]
    tunnel: w93 -> [w287]
    tunnel: [w289] -> w89
    timing: w6 -> [_]
    timing-out: [_] -> w5
    tunnel: w2 -> [w273]
    tunnel: w1 -> [w272]
    stop <- w290 stop-if-true
    n102 = node-c288() -> ()  [unwired: 1 in, 1 out]
    n103 = local read "OUT cOPF"() -> (w275:T1)
    n104 = Flatten To JSON(anything=w275, error in (no error)=w287) -> (JSON string=w276:string, 11:w274:errorcluster)  [unwired: 1 in]
    n105 = UDP Write(address=w273, port or service name=w272, connection ID=w288, data in=w276, 8:w274) -> (error out=w285:errorcluster, 3:w286:refnum<k16>)  [unwired: 1 in]
    n106 = UDP Read(connection ID=w286, max size (548)=4000, timeout ms (25000)=20, 8:w285) -> (data out=w294:string, error out=w293:errorcluster, 3:w284:refnum<k16>)  [unwired: 2 out]
    n107 = call <vilib>:"Is Empty.vi"("JSON"=w294) -> ("Empty"=w292:bool)  [unwired: 4 in]
    n108 = Not(x=w292) -> (.not. x?=→"cOPF data":bool)
    n109 = case shown="False" w292 {
      tunnel: w293 -> [w299 w303]
      tunnel: w294 -> [_ w302]
      tunnel: [w299 w304] -> w289
      tunnel: [w298 w300] -> w283
      frame True {
        (unwired) FALSE ("Found")
        n110 = local read "IN cOPF"() -> (w298:T1)
      }
      frame False {
        n111 = Unflatten From JSON(JSON string=w302, type and defaults=T1 {"Info"={"Resource"="Zenone", "Problem"=0.0, "Timestamp"=0.0}, "Data"={"Operation_mode"="Grid connected", "solution_feasible"=0.0, "Optimal_slack"="AFE 1", "setpoints"=[], "upper_layer_grid_info"={"Frequency"=0.0, "Angle"=0.0, "Magnitude"=0.0}, "SC_soc"=0.0, "PV"={"perun"=0.0, "solarmax"=0.0, "facade"=0.0, "emul4"=0.0, "emul5"=0.0, "emul6"=0.0, "emul7"=0.0}, "P_pv_facade"=0.0}} ("IN iOPF"), error in (no error)=w303) -> (value=w300:T1, error out=w304:errorcluster)  [unwired: 4 in]
      }
    }
    n112 = Unbundle By Name(w283) -> ("Info.Timestamp"=w277:dbl, "Data.setpoints"=w282:dbl[])
    n113 = local write "IN cOPF"(w283) -> ()
    n114 = local read "Stop"() -> (w290:bool)
    n115 = To Time Stamp(1:w277) -> (0:→"time connected":timestamp)
    n116 = Index Array(array=w282, index=10) -> (element=→"P_bess_connected":dbl)
    n117 = node-c288() -> ()  [unwired: 1 in, 1 out]
  }
  n118 = while {
    tunnel: w87 -> [w329]
    tunnel: w86 -> [w328]
    shift-right: [w313] -> w92
    shift-left: w100 -> [w318]
    tunnel: w99 -> [w315]
    tunnel: [w319] -> w91
    stop <- w322 stop-if-true
    n119 = local read "OUT iOPF"() -> (w320:T1)
    n120 = Wait (ms)(milliseconds to wait=u32 100) -> ()  [unwired: 1 out]
    n121 = Flatten To JSON(anything=w320, error in (no error)=w315) -> (JSON string=w321:string, 11:w314:errorcluster)  [unwired: 1 in]
    n122 = UDP Write(address=w328, port or service name=w329, connection ID=w318, data in=w321, 8:w314) -> (error out=w316:errorcluster, 3:w317:refnum<k16>)  [unwired: 1 in]
    n123 = UDP Read(connection ID=w317, max size (548)=4000, timeout ms (25000)=500, 8:w316) -> (data out=w312:string, error out=w326:errorcluster, 3:w313:refnum<k16>)  [unwired: 2 out]
    n124 = call <vilib>:"Is Empty.vi"("JSON"=w312) -> ("Empty"=w325:bool)  [unwired: 4 in]
    n125 = Not(x=w325) -> (.not. x?=→"iOPF data":bool)
    n126 = case shown="False" w325 {
      tunnel: w326 -> [w331 w333]
      tunnel: [w330 w336] -> w308
      tunnel: w312 -> [_ w332]
      tunnel: [w331 w335] -> w319
      frame True {
        (unwired) FALSE ("Found")
        n127 = local read "IN iOPF"() -> (w330:T1)
      }
      frame False {
        n128 = Unflatten From JSON(JSON string=w332, type and defaults=T1 {"Info"={"Resource"="Zenone", "Problem"=0.0, "Timestamp"=0.0}, "Data"={"Operation_mode"="Grid connected", "solution_feasible"=0.0, "Optimal_slack"="AFE 1", "setpoints"=[], "upper_layer_grid_info"={"Frequency"=0.0, "Angle"=0.0, "Magnitude"=0.0}, "SC_soc"=0.0, "PV"={"perun"=0.0, "solarmax"=0.0, "facade"=0.0, "emul4"=0.0, "emul5"=0.0, "emul6"=0.0, "emul7"=0.0}, "P_pv_facade"=0.0}} ("IN cOPF"), error in (no error)=w333) -> (value=w336:T1, error out=w335:errorcluster)  [unwired: 4 in]
      }
    }
    n129 = Unbundle By Name(w308) -> ("Info.Timestamp"=w306:dbl, "Data.setpoints"=w311:dbl[])
    n130 = local write "IN iOPF"(w308) -> ()
    n131 = local read "Stop"() -> (w322:bool)
    n132 = Index Array(array=w311, index=10) -> (element=→"P_bess_island":dbl)
    n133 = To Time Stamp(1:w306) -> (0:→"time island":timestamp)
  }
  n134 = while {
    tunnel: w27 -> [w344]
    tunnel: [w339] -> w26
    shift-right: [w338] -> w25
    shift-left: w28 -> [w345]
    stop <- w337 stop-if-true
    n135 = UDP Read(connection ID=w345, 8:w344) -> (data out=w342:string, error out=w340:errorcluster, 3:w338:refnum<k16>)  [unwired: 2 in, 2 out]
    n136 = call <vilib>:"Is Empty.vi"("JSON"=w342) -> ("Empty"=w343:bool)  [unwired: 4 in]
    n137 = case shown="False" w343 {
      tunnel: w342 -> [_ w352]
      tunnel: [w347 w350] -> w341
      tunnel: w340 -> [w346 w349]
      tunnel: [w346 w348] -> w339
      frame True {
        n138 = local read "IN Meteo"() -> (w347:T9)
      }
      frame False {
        n139 = Unflatten From JSON(JSON string=w352, type and defaults=T9 {"Info"={"Resource"="MeteoBox", "Problem"=FALSE, "Timestamp"=0.0}, "Data"={"GI"=0.0, "GHI"=0.0, "GVI"=0.0, "Tair"=0.0, "Tcell roof"=0.0, "Global_Total_Irr"=0.0, "Diffused_Irr"=0.0, "Tcell facade"=0.0, "PV_mpp"={"perun"=0.0, "solarmax"=0.0, "facade"=0.0, "emul4"=0.0, "emul5"=0.0, "emul6"=0.0, "emul7"=0.0}}} ("Cluster"), error in (no error)=w349) -> (value=w350:T9, error out=w348:errorcluster)  [unwired: 4 in]
      }
    }
    n140 = local write "IN Meteo"(w341) -> ()
    n141 = local read "Stop"() -> (w337:bool)
  }
  n142 = Initialize Array(FALSE, "nb instances") -> (w112:bool[])
  n143 = Initialize Array(FALSE, "nb instances") -> (w110:bool[])
  n144 = String To IP(1:w42) -> (0:w41:u32)
  n145 = String To IP(1:w46) -> (0:w47:u32)
  n146 = UDP Open(7:w47, 9:200 ("timeout ms (25000)"), 11:w44) -> (port=w43:refnum<k16>, 0:w34:errorcluster)  [unwired: 2 in, 1 out]
  n147 = while {
    tunnel: [w359] -> w48
    tunnel: w41 -> [w369]
    tunnel: w40 -> [w368]
    tunnel: w34 -> [w363]
    shift-right: [w358] -> w33
    shift-left: w43 -> [w370]
    stop <- w366 stop-if-true
    # "Central data aquisition"
    n148 = local read "Zenone_Q"() -> (w364:dbl)
    n149 = local read "Zenone_P"() -> (w365:dbl)
    n150 = local read "setpoints"() -> (w372:dbl[])
    n151 = Wait (ms)(milliseconds to wait=u32 100) -> ()  [unwired: 1 out]
    n152 = call "Setpoint.vi"("ZENONE.Q_set [kVAr]"=w364, "ZENONE.P_set [kW]"=w365, "setpoints IN"=w372) -> ("OUT"=w353:T7)  [unwired: 8 in]
    n153 = Flatten To JSON(anything=w353) -> (JSON string=w371:string)  [unwired: 2 in, 1 out]
    n154 = case shown="False" "Send sp AC?" {
      tunnel: w371 -> [_ w397]
      tunnel: w370 -> [w390 w396]
      tunnel: w369 -> [_ w395]
      tunnel: w368 -> [_ w394]
      tunnel: [w390 w393] -> w361
      tunnel: [w389 w392] -> w360
      tunnel: w363 -> [w389 w391]
      frame False {
      }
      frame True {
        n155 = UDP Write(address=w395, port or service name=w394, connection ID=w396, data in=w397, 8:w391) -> (error out=w392:errorcluster, 3:w393:refnum<k16>)  [unwired: 1 in]
      }
    }
    n156 = UDP Read(connection ID=w361, max size (548)=2000, 8:w360) -> (data out=w356:string, error out=w357:errorcluster, 3:w358:refnum<k16>)  [unwired: 1 in, 2 out]
    n157 = call <vilib>:"Is Empty.vi"("JSON"=w356) -> ("Empty"=w355:bool)  [unwired: 4 in]
    n158 = case shown="False" w355 {
      tunnel: [w373 w380] -> w359
      tunnel: w356 -> [_ w379]
      tunnel: w357 -> [w373 w375]
      frame True {
      }
      frame False {
        n159 = call <vilib>:"Find Item.vi"("$Path or Item Name"="Facade", "JSON"=w379) -> ("<JSON>"=w377:string, "Found"=w376:bool)  [unwired: 6 in, 2 out]
        n160 = case shown="False" w376 {
          tunnel: w377 -> [_ w388]
          tunnel: w375 -> [w382 w387]
          tunnel: [w382 w386] -> w380
          tunnel: [w381 w383] -> w374
          frame False {
            n161 = local read "P_pv_facade"() -> (w381:dbl)
          }
          frame True {
            n162 = Unflatten From JSON(JSON string=w388, type and defaults=T31 {"Info"={"Resource"="Zenone", "Problem"=FALSE, "Timestamp"=0.0}, "Data"={"P"=0.0, "Q"=0.0, "Pset"=0.0, "Qset"=0.0}} ("Cluster"), error in (no error)=w387) -> (value=w384:T31, error out=w386:errorcluster)  [unwired: 4 in]
            n163 = Unbundle By Name(w384) -> ("Data.P"=w383:dbl)
          }
        }
        n164 = local write "P_pv_facade"(w374) -> ()
      }
    }
    n165 = local read "Stop"() -> (w366:bool)
  }
  n166 = node-c288() -> (w107:T28)  [unwired: 4 in]
  n167 = timed-loop {
    shift-right: [w419] -> _
    shift-left: w112 -> [w420]
    shift-right: [w417] -> _
    shift-left: w110 -> [w418]
    tunnel: "nb instances" -> [w416]
    shift-right: [w409] -> _
    shift-left: State_Machine."Grid connected" ("State") -> [w410]
    timing: w107 -> [_]
    timing-out: [_] -> w106
    shift-right: [w399] -> _
    shift-left: errorcluster {"status"=FALSE, "code"=0, "source"=""} ("error constant") -> [w400]
    stop <- "Stop" stop-if-true
    # "State Machine While Loop"
    n168 = node-c288() -> (→"Iteration Duration":dbl)  [unwired: 1 in, 2 out]
    n169 = case "State Machine Case Structure" shown="\"Grid connected\", Default" w410 {
      tunnel: "IN synchro" -> [w452 w551 w661 w776 w900]
      tunnel: "IN AFE" -> [w451 w552 w662 w777 w899]
      tunnel: "IN cOPF" -> [w450 w553 w663 w778 w898]
      tunnel: "IN iOPF" -> [w449 w554 w664 w779 w897]
      tunnel: w420 -> [w448 w550 w660 w775 w896]
      tunnel: [w448 w549 w660 w775 w896] -> w419
      tunnel: w418 -> [w447 w548 w659 w774 w895]
      tunnel: [w447 w547 w659 w774 w895] -> w417
      tunnel: w416 -> [_ w546 _ _ _]
      tunnel: [w443 w538 w655 w770 w891] -> w415
      tunnel: [w445 w540 w656 w771 w892] -> w414
      tunnel: [w444 w539 w657 w772 w893] -> w413
      tunnel: [w446 w541 w658 w773 w894] -> w412
      tunnel: [w431 w527 w645 w758 w879] -> w409
      tunnel: "IN PV+SC" -> [w437 w531 w649 w763 w884]
      tunnel: [w436 w528 w646 w760 w881] -> w403
      tunnel: "IN Meteo" -> [w430 w524 w643 w756 w875]
      tunnel: "SCADA" -> [_ _ w640 w754 w871]
      tunnel: w400 -> [w427 w520 w635 w750 w866]
      tunnel: [w425 w518 w633 w749 w864] -> w399
      frame "Grid connected", Default {
        # "Grid connected - Display a dialog box with a message specific to State 1, then go back to the Wait for Event state."
        n170 = flat-sequence {
          tunnel: w452 -> [w478]
          tunnel: w451 -> [w479]
          tunnel: w450 -> [w477]
          tunnel: w449 -> [w476]
          tunnel: [w479] -> w442
          tunnel: [w478] -> w441
          tunnel: [w477] -> w440
          tunnel: [w476] -> w439
          tunnel: [w461] -> w438
          tunnel: w437 -> [w469]
          tunnel: [w475] -> w435
          tunnel: [w469] -> w434
          tunnel: [w461] -> w433
          tunnel: w430 -> [w465]
          tunnel: [w464] -> w429
          tunnel: [w462] -> w428
          tunnel: w427 -> [w462]
          tunnel: w442 -> [w511]
          tunnel: w441 -> [w510]
          tunnel: w440 -> [w509]
          tunnel: w439 -> [w508]
          tunnel: w438 -> [w506]
          tunnel: w435 -> [w505]
          tunnel: w434 -> [w503]
          tunnel: w433 -> [w500]
          tunnel: [w515] -> w446
          tunnel: [w514] -> w445
          tunnel: [w513] -> w444
          tunnel: [w512] -> w443
          tunnel: [w504] -> w436
          tunnel: w429 -> [w492]
          tunnel: [w488] -> w426
          tunnel: w428 -> [w488]
          frame #0 {
            # "from island OPF"
            # "from connected OPF"
            # "from resource"
            # "from synchrocheck"
            n171 = Unbundle By Name(w469) -> ("Data.Forming/Following"=→"forming SC?":bool, "Data.measurements SC.SOC"=w466:dbl)
            n172 = Unbundle By Name(w478) -> ("Data.Synchronised?"=→"synchronised?":bool, "Data.V_UpStream"=w468:T25, "Data.V_Downstream"=w467:T25)
            n173 = Unbundle By Name(w465) -> ("Data.PV_mpp"=w464:T36)
            n174 = Unbundle By Name(w479) -> ("Data.Forming/Following"=w484:bool[])
            n175 = Unbundle By Name(w477) -> ("Data.solution_feasible"=w472:dbl, "Data.setpoints"=w459:dbl[])
            n176 = Unbundle By Name(w476) -> ("Data.solution_feasible"=w474:dbl)
            n177 = local write "to connected-island"(FALSE ("to connected island")) -> ()
            n178 = local write "to grid connection"(TRUE ("to grid connection")) -> ()
            n179 = local write "to prepare for island"(FALSE ("to prepare for island")) -> ()
            n180 = local write "to island"(FALSE ("to island")) -> ()
            n181 = local write "to prepare for grid connection"(FALSE ("to prepare for grid connection")) -> ()
            n182 = local read "old_sp_island"() -> (w458:dbl[])
            n183 = local read "old_sp_island_bool"() -> (w460:bool)
            n184 = Not Equal To 0?(x=w472) -> (x != 0?=→"cOPF valid?":bool)
            n185 = Not Equal To 0?(x=w474) -> (x != 0?=→"iOPF valid":bool)
            n186 = local write "setpoints"(w459) -> ()
            n187 = Or Array Elements(Boolean array=w484) -> (logical OR=→"forming AFE?":bool)
            n188 = local write "SC_soc"(w466) -> ()
            n189 = call "up_grid_data.vi"("Data.V_Downstream"=w467, "Data.V_UpStream"=w468) -> ("upper layer grid info"=w475:T35)  [unwired: 5 in, 4 out]
            n190 = Select(t=w458, s=w460, f=w459) -> (s? t:f=w461:dbl[])
          }
          frame #1 {
            # "send to island OPF"
            # "send to resource"
            # "send to connected OPF"
            # "send to synchrocheck"
            n191 = local read "P_pv_facade"() -> (w489:dbl)
            n192 = local read "SC_soc"() -> (w494:dbl)
            n193 = local read "SC_soc"() -> (w493:dbl)
            n194 = call "distribute_setpoints.vi"("setpoints"=w506, "upper layer grid info"=w505) -> ("references"=w507:T21)  [unwired: 9 in]
            n195 = call "distribute_setpoints_DC.vi"("setpoints"=w500) -> ("reference_DC"=w501:T17)  [unwired: 10 in]
            n196 = Bundle By Name(cluster=w509, "Data.Operation_mode"="Grid connected" ("Operation_mode"), "Data.upper_layer_grid_info"=w505, "Data.SC_soc"=w494, "Data.P_pv_facade"=w489, "Data.PV"=w492) -> (w513:T1)
            n197 = Bundle By Name(cluster=w508, "Data.Operation_mode"="Grid connected" ("Operation_mode"), "Data.upper_layer_grid_info"=w505, "Data.SC_soc"=w493, "Data.P_pv_facade"=w489, "Data.PV"=w492) -> (w515:T1)
            n198 = Bundle By Name(cluster=w503, "Data.Start following"=TRUE, "Data.Start forming"=FALSE, "Data.SC references"=w501) -> (w504:T12)
            n199 = Bundle By Name(cluster=w510, "Data.close/open relay"=TRUE, "Data.Operation mode"="Grid connected" ("Operation_mode")) -> (w512:T22)
            n200 = Bundle By Name(cluster=w511, "Data.Start forming 2"=FALSE, "Data.Start following 2"=TRUE, "Data.Start following 1"=TRUE, "Data.Start forming 1"=FALSE, "Data.references"=w507) -> (w514:T18)
            n201 = local write "old_sp_island_bool"(FALSE ("old_sp_island_bool")) -> ()
          }
        }
        n202 = case shown="True" "to prepare for island" {
          tunnel: [State_Machine."Grid connected" ("State") State_Machine."Prepare for island" ("State")] -> w431
          tunnel: [w453 w455] -> w425
          tunnel: w426 -> [w453 w455]
          frame False {
          }
          frame True {
            n203 = local write "Reset_magnitude"(TRUE ("Rest_PI_V")) -> ()
          }
        }
      }
      frame "Prepare for island" {
        n204 = flat-sequence {
          tunnel: w554 -> [w585]
          tunnel: w553 -> [w584]
          tunnel: w552 -> [w582]
          tunnel: w551 -> [w583]
          tunnel: w550 -> [w594]
          tunnel: w548 -> [w592]
          tunnel: w546 -> [w588]
          tunnel: [w593] -> w545
          tunnel: [w591] -> w544
          tunnel: [w590] -> w543
          tunnel: [w589] -> w542
          tunnel: [w585] -> w537
          tunnel: [w584] -> w536
          tunnel: [w583] -> w535
          tunnel: [w582] -> w534
          tunnel: [w574] -> w533
          tunnel: [w581] -> w532
          tunnel: w531 -> [w575]
          tunnel: [w575] -> w530
          tunnel: [w574] -> w529
          tunnel: w524 -> [w566]
          tunnel: [w565] -> w523
          tunnel: [w563] -> w521
          tunnel: w520 -> [w563]
          tunnel: w545 -> [w631]
          tunnel: w544 -> [w630]
          tunnel: w543 -> [w610]
          tunnel: w542 -> [w611]
          tunnel: w537 -> [w621]
          tunnel: w536 -> [w620]
          tunnel: w535 -> [w619]
          tunnel: w534 -> [w618]
          tunnel: w533 -> [w616]
          tunnel: w532 -> [w605]
          tunnel: w530 -> [w615]
          tunnel: w529 -> [w612]
          tunnel: [w631] -> w549
          tunnel: [w630] -> w547
          tunnel: [w625] -> w541
          tunnel: [w624] -> w540
          tunnel: [w623] -> w539
          tunnel: [w622] -> w538
          tunnel: [w614] -> w528
          tunnel: [w611] -> w526
          tunnel: [w610] -> w525
          tunnel: w523 -> [w600]
          tunnel: [w596] -> w519
          tunnel: w521 -> [w596]
          frame #0 {
            # "from island OPF"
            # "from connected OPF"
            # "from resource"
            # "from synchrocheck"
            n205 = Unbundle By Name(w566) -> ("Data.PV_mpp"=w565:T36)
            n206 = Unbundle By Name(w575) -> ("Data.Forming/Following"=w576:bool, "Data.measurements SC.SOC"=w567:dbl)
            n207 = Unbundle By Name(w584) -> ("Data.solution_feasible"=w578:dbl, "Data.setpoints"=w574:dbl[])
            n208 = Unbundle By Name(w582) -> ("Data.Forming/Following"=w595:bool[])
            n209 = Unbundle By Name(w585) -> ("Data.solution_feasible"=w579:dbl)
            n210 = Unbundle By Name(w583) -> ("Data.Synchronised?"=w587:bool, "Data.V_UpStream"=w569:T25, "Data.V_Downstream"=w568:T25)
            n211 = local write "to connected-island"(FALSE ("to connected island")) -> ()
            n212 = local write "to grid connection"(FALSE ("to grid connection")) -> ()
            n213 = local write "to prepare for island"(TRUE ("to prepare for island")) -> ()
            n214 = local write "to island"(FALSE ("to island")) -> ()
            n215 = local write "to prepare for grid connection"(FALSE ("to prepare for grid connection")) -> ()
            n216 = local write "synchronised?"(w587) -> ()
            n217 = Or Array Elements(Boolean array=w595) -> (logical OR=w586:bool)
            n218 = local write "setpoints"(w574) -> ()
            n219 = local write "forming SC?"(w576) -> ()
            n220 = local write "SC_soc"(w567) -> ()
            n221 = Not Equal To 0?(x=w578) -> (x != 0?=w577:bool)
            n222 = Not Equal To 0?(x=w579) -> (x != 0?=w580:bool)
            n223 = local write "forming AFE?"(w586) -> ()
            n224 = call "check multiple instances.vi"("nb instances"=w588, "array elements in"=w594, "new element"=w577) -> ("array elements out"=w593:bool[], "out"=w589:bool)  [unwired: 7 in]
            n225 = local write "cOPF valid?"(w577) -> ()
            n226 = call "check multiple instances.vi"("nb instances"=w588, "array elements in"=w592, "new element"=w580) -> ("array elements out"=w591:bool[], "out"=w590:bool)  [unwired: 7 in]
            n227 = local write "iOPF valid"(w580) -> ()
            n228 = call "up_grid_data.vi"("Data.V_Downstream"=w568, "Data.V_UpStream"=w569) -> ("upper layer grid info"=w581:T35)  [unwired: 5 in, 4 out]
          }
          frame #1 {
            # "send to island OPF"
            # "send to resource"
            # "send to connected OPF"
            # "send to synchrocheck"
            n229 = local read "P_pv_facade"() -> (w597:dbl)
            n230 = local read "optimal_slack"() -> (w628:string)
            n231 = local read "optimal_slack"() -> (w629:string)
            n232 = call "distribute_setpoints_DC.vi"("setpoints"=w612) -> ("reference_DC"=w604:T17)  [unwired: 10 in]
            n233 = call "distribute_setpoints.vi"("setpoints"=w616, "upper layer grid info"=w605) -> ("references"=w617:T21)  [unwired: 9 in]
            n234 = local read "SC_soc"() -> (w602:dbl)
            n235 = local read "SC_soc"() -> (w601:dbl)
            n236 = Bundle By Name(cluster=w620, "Data.Operation_mode"="Prepare Island" ("Operation_mode"), "Data.Optimal_slack"=w628, "Data.upper_layer_grid_info"=w605, "Data.SC_soc"=w602, "Data.P_pv_facade"=w597, "Data.PV"=w600) -> (w623:T1)
            n237 = Bundle By Name(cluster=w621, "Data.Operation_mode"="Prepare Island" ("Operation_mode"), "Data.Optimal_slack"=w629, "Data.upper_layer_grid_info"=w605, "Data.SC_soc"=w601, "Data.P_pv_facade"=w597, "Data.PV"=w600) -> (w625:T1)
            n238 = Bundle By Name(cluster=w619, "Data.close/open relay"=TRUE, "Data.Operation mode"="Prepare Island" ("Operation_mode")) -> (w622:T22)
            n239 = Bundle By Name(cluster=w618, "Data.Start forming 2"=FALSE, "Data.Start following 2"=TRUE, "Data.Start following 1"=TRUE, "Data.Start forming 1"=FALSE, "Data.references"=w617) -> (w624:T18)
            n240 = Bundle By Name(cluster=w615, "Data.Start following"=TRUE, "Data.Start forming"=FALSE, "Data.SC references"=w604) -> (w614:T12)
          }
        }
        n241 = disable-structure shown="Disabled" {
          disable-tunnel: [w558 _] -> _
          disable-tunnel: "to connected-island" -> [w557 _]
          disable-tunnel: w526 -> [w556 _]
          disable-tunnel: w525 -> [w555 _]
          frame Disabled {
            n242 = Compound Arithmetic op=AND(w556, w555, w557) -> (w558:bool)
          }
          frame Enabled {
          }
        }
        n243 = case shown="False" "to connected-island" {
          tunnel: [State_Machine."Prepare for island" ("State") State_Machine."Forming but connected" ("State")] -> w527
          tunnel: [w559 w561] -> w518
          tunnel: w519 -> [w559 w561]
          frame False {
          }
          frame True {
            # "only go to next state if OPFs are feasible for 7 timesteps"
          }
        }
      }
      frame "Forming but connected" {
        # "Island - Display a dialog box with a message specific to State 3, then go back to the Wait for Event state."
        n244 = flat-sequence {
          tunnel: w664 -> [w698]
          tunnel: w663 -> [w697]
          tunnel: w662 -> [w673]
          tunnel: w661 -> [w696]
          tunnel: [w698] -> w654
          tunnel: [w697] -> w653
          tunnel: [w696] -> w652
          tunnel: [w676] -> w651
          tunnel: [w681] -> w650
          tunnel: w649 -> [w690]
          tunnel: [w690] -> w648
          tunnel: [w676] -> w647
          tunnel: [w687] -> w644
          tunnel: w643 -> [w685]
          tunnel: [w684] -> w642
          tunnel: w640 -> [w682]
          tunnel: [w680] -> w639
          tunnel: [w677] -> w638
          tunnel: ["Reset_magnitude"] -> w637
          tunnel: [w674] -> w636
          tunnel: w635 -> [w674]
          tunnel: [w673] -> w632
          tunnel: w654 -> [w725]
          tunnel: w653 -> [w740]
          tunnel: w652 -> [w739]
          tunnel: w651 -> [w737]
          tunnel: w650 -> [w720]
          tunnel: w648 -> [w736]
          tunnel: w647 -> [w733]
          tunnel: [w744] -> w658
          tunnel: [w743] -> w657
          tunnel: [w742] -> w656
          tunnel: [w741] -> w655
          tunnel: [w735] -> w646
          tunnel: w644 -> [_]
          tunnel: w642 -> [w724]
          tunnel: w639 -> [w718]
          tunnel: w638 -> [w717]
          tunnel: w637 -> [w712]
          tunnel: [w708] -> w634
          tunnel: w636 -> [w708]
          tunnel: w632 -> [w707]
          frame #0 {
            # "from island OPF"
            # "from connected OPF"
            # "from resource"
            # "from synchrocheck"
            n245 = Unbundle By Name(w690) -> ("Data.Forming/Following"=w691:bool, "Data.measurements SC.SOC"=w686:dbl)
            n246 = Unbundle By Name(w698) -> ("Data.solution_feasible"=w695:dbl, "Data.upper_layer_grid_info"=w687:T35)  [unwired: 1 out]
            n247 = Unbundle By Name(w673) -> ("Data.Forming/Following"=w705:bool[])
            n248 = Unbundle By Name(w697) -> ("Data.solution_feasible"=w694:dbl, "Data.setpoints"=w676:dbl[])
            n249 = Unbundle By Name(w696) -> ("Data.Synchronised?"=w700:bool, "Data.V_UpStream"=w689:T25, "Data.V_Downstream"=w688:T25)
            n250 = Unbundle By Name(w682) -> ("Data.Voltage mag"=w679:dbl[])
            n251 = Unbundle By Name(w685) -> ("Data.PV_mpp"=w684:T36)
            n252 = local write "to connected-island"(TRUE ("to prepare for grid connection")) -> ()
            n253 = local write "to prepare for grid connection"(FALSE ("to prepare for grid connection")) -> ()
            n254 = local write "to grid connection"(FALSE ("to grid connection")) -> ()
            n255 = local write "to prepare for island"(FALSE ("to prepare for island")) -> ()
            n256 = local write "to island"(FALSE ("to island")) -> ()
            n257 = local write "synchronised?"(w700) -> ()
            n258 = Not Equal To 0?(x=w694) -> (x != 0?=w693:bool)
            n259 = local write "setpoints"(w676) -> ()
            n260 = Not Equal To 0?(x=w695) -> (x != 0?=w692:bool)
            n261 = Or Array Elements(Boolean array=w705) -> (logical OR=w699:bool)
            n262 = local write "forming SC?"(w691) -> ()
            n263 = Index Array(array=w679, index=18) -> (element=w677:dbl)
            n264 = local write "SC_soc"(w686) -> ()
            n265 = local write "forming AFE?"(w699) -> ()
            n266 = local write "cOPF valid?"(w693) -> ()
            n267 = call "up_grid_data.vi"("Data.V_Downstream"=w688, "Data.V_UpStream"=w689) -> ("upper layer grid info"=w681:T35)  [unwired: 5 in, 4 out]
            n268 = local write "iOPF valid"(w692) -> ()
            n269 = Unbundle By Name(w681) -> ("Magnitude"=w680:dbl)
          }
          frame #1 {
            # "send to island OPF"
            # "send to connected OPF"
            # "send to resource"
            # "send to synchrocheck"
            n270 = call <userlib>:"Boolean Trigger__ogtk.vi"("Boolean Input"=w712) -> ("Rising Edge"=w711:bool)  [unwired: 1 in, 1 out]
            n271 = call "PID2_2V.vi"("reinitialize? (F)"=w711, "V_afe"=w717, "V_up"=w718) -> ("output"=w706:dbl)  [unwired: 8 in]
            "V_control" <- w706
            n272 = Unbundle(w720) -> ("Frequency"=w716:dbl)  [unwired: 2 out]
            "V_freq" <- w716
            n273 = local read "optimal_slack"() -> (w748:string)
            n274 = local read "P_pv_facade"() -> (w721:dbl)
            n275 = local read "optimal_slack"() -> (w747:string)
            n276 = call "distribute_setpoints_DC.vi"("setpoints"=w733) -> ("reference_DC"=w729:T17)  [unwired: 10 in]
            n277 = local read "SC_soc"() -> (w726:dbl)
            n278 = local read "SC_soc"() -> (w727:dbl)
            n279 = Bundle(cluster=T35 {"Frequency"=0.0, "Angle"=0.0, "Magnitude"=0.0} ("upper layer grid info"), "Frequency"=w716, "Angle"=0.0, "Magnitude"=w706) -> (w732:T35)
            n280 = Bundle("output"=w706) -> (→"V control":cluster{"output":dbl})  [unwired: 1 in]
            n281 = call "distribute_setpoints.vi"("setpoints"=w737, "upper layer grid info"=w732) -> ("references"=w738:T21)  [unwired: 9 in]
            n282 = Bundle By Name(cluster=w740, "Data.Operation_mode"=T34 "Forming but connected" ("Operation_mode"), "Data.Optimal_slack"=w747, "Data.upper_layer_grid_info"=w720, "Data.SC_soc"=w727, "Data.P_pv_facade"=w721, "Data.PV"=w724) -> (w743:T1)
            n283 = Bundle By Name(cluster=w725, "Data.Operation_mode"=T34 "Forming but connected" ("Operation_mode"), "Data.Optimal_slack"=w748, "Data.upper_layer_grid_info"=w720, "Data.SC_soc"=w726, "Data.P_pv_facade"=w721, "Data.PV"=w724) -> (w744:T1)
            n284 = Bundle By Name(cluster=w736, "Data.Start following"=FALSE, "Data.Start forming"=TRUE, "Data.SC references"=w729) -> (w735:T12)
            n285 = Bundle By Name(cluster=w739, "Data.close/open relay"=TRUE, "Data.Operation mode"=T34 "Forming but connected" ("Operation_mode")) -> (w741:T22)
            n286 = Bundle By Name(cluster=w707, "Data.Start forming 2"=FALSE, "Data.Start following 2"=TRUE, "Data.Start following 1"=FALSE, "Data.Start forming 1"=TRUE, "Data.references"=w738) -> (w742:T18)
            n287 = local write "Reset_magnitude"(FALSE ("Rest_PI_V")) -> ()
            "V_upstream" <- w718
            "V_afe" <- w717
          }
        }
        n288 = case shown="True" "to island" {
          tunnel: [State_Machine."Forming but connected" ("State") State_Machine."Island" ("State")] -> w645
          tunnel: w634 -> [w665 w668]
          tunnel: [w665 w668] -> w633
          frame False {
          }
          frame True {
            # "only go to next state if OPFs are feasible\n for 7 timesteps"
            n289 = local read "V_control"() -> (→"V_control_fix_for_island":dbl)
            n290 = local read "V_freq"() -> (→"V_freq_for_island":dbl)
            n291 = local write "Reset_magnitude"(TRUE ("Rest_PI_V")) -> ()
            n292 = local write "delta angle"(0.0 ("delta angle")) -> ()
          }
        }
      }
      frame "Island" {
        # "Island - Display a dialog box with a message specific to State 3, then go back to the Wait for Event state."
        n293 = flat-sequence {
          tunnel: w779 -> [w812]
          tunnel: w778 -> [w811]
          tunnel: w777 -> [w810]
          tunnel: w776 -> [w809]
          tunnel: [w812] -> w769
          tunnel: [w811] -> w768
          tunnel: [w810] -> w767
          tunnel: [w809] -> w766
          tunnel: [w802] -> w765
          tunnel: [w793] -> w764
          tunnel: w763 -> [w803]
          tunnel: [w803] -> w762
          tunnel: [w802] -> w761
          tunnel: [w799] -> w757
          tunnel: w756 -> [w797]
          tunnel: [w796] -> w755
          tunnel: w754 -> [w794]
          tunnel: [w792] -> w753
          tunnel: [w788] -> w752
          tunnel: [w787] -> w751
          tunnel: w769 -> [w833]
          tunnel: w768 -> [w852]
          tunnel: w767 -> [w851]
          tunnel: w766 -> [w850]
          tunnel: w765 -> [w848]
          tunnel: w764 -> [w827]
          tunnel: w762 -> [w847]
          tunnel: w761 -> [w844]
          tunnel: [w856] -> w773
          tunnel: [w855] -> w772
          tunnel: [w854] -> w771
          tunnel: [w853] -> w770
          tunnel: [w846] -> w760
          tunnel: w757 -> [_]
          tunnel: w755 -> [w832]
          tunnel: w753 -> [w825]
          tunnel: w752 -> [w824]
          tunnel: w751 -> [w826]
          frame #0 {
            # "from island OPF"
            # "from connected OPF"
            # "from resource"
            # "from synchrocheck"
            n294 = Unbundle By Name(w803) -> ("Data.Forming/Following"=w804:bool, "Data.measurements SC.SOC"=w798:dbl)
            n295 = Unbundle By Name(w812) -> ("Data.solution_feasible"=w808:dbl, "Data.setpoints"=w802:dbl[], "Data.upper_layer_grid_info"=w799:T35)
            n296 = Unbundle By Name(w810) -> ("Data.Forming/Following"=w819:bool[])
            n297 = Unbundle By Name(w811) -> ("Data.solution_feasible"=w807:dbl)
            n298 = Unbundle By Name(w809) -> ("Data.Synchronised?"=w814:bool, "Data.V_UpStream"=w801:T25, "Data.V_Downstream"=w800:T25)
            n299 = Unbundle By Name(w794) -> ("Data.Voltage mag"=w791:dbl[])  [unwired: 1 out]
            n300 = Unbundle By Name(w797) -> ("Data.PV_mpp"=w796:T36)
            n301 = local write "to connected-island"(FALSE ("to connected island")) -> ()
            n302 = local write "to grid connection"(FALSE ("to grid connection")) -> ()
            n303 = local write "to prepare for island"(FALSE ("to prepare for island")) -> ()
            n304 = local write "to island"(TRUE ("to island")) -> ()
            n305 = local write "to prepare for grid connection"(FALSE ("to prepare for grid connection")) -> ()
            n306 = local write "synchronised?"(w814) -> ()
            n307 = Not Equal To 0?(x=w807) -> (x != 0?=w806:bool)
            n308 = local write "setpoints"(w802) -> ()
            n309 = Not Equal To 0?(x=w808) -> (x != 0?=w805:bool)
            n310 = Or Array Elements(Boolean array=w819) -> (logical OR=w813:bool)
            n311 = local write "forming SC?"(w804) -> ()
            n312 = Index Array(array=w791, index #1=14 ("index"), index #2=18 ("index")) -> (element #2=w788:dbl)  [unwired: 1 out]
            n313 = local write "SC_soc"(w798) -> ()
            n314 = local write "forming AFE?"(w813) -> ()
            n315 = local write "cOPF valid?"(w806) -> ()
            n316 = local write "iOPF valid"(w805) -> ()
            n317 = local read "Reset_magnitude"() -> (w787:bool)
            n318 = call "up_grid_data.vi"("Data.V_Downstream"=w800, "Data.V_UpStream"=w801) -> ("upper layer grid info"=w793:T35)  [unwired: 5 in, 4 out]
            n319 = Unbundle By Name(w793) -> ("Magnitude"=w792:dbl)
          }
          frame #1 {
            (unwired) 230.0 ("Magnitude")
            # "send to island OPF"
            # "send to connected OPF"
            # "send to resource"
            # "send to synchrocheck"
            n320 = local read "V_control_fix_for_island"() -> (w821:dbl)
            n321 = Unbundle(w827) -> ()  [unwired: 3 out]
            n322 = call <userlib>:"Boolean Trigger__ogtk.vi"("Boolean Input"=w826) -> ()  [unwired: 1 in, 2 out]
            n323 = local read "optimal_slack"() -> (w860:string)
            n324 = local read "P_pv_facade"() -> (w828:dbl)
            n325 = local read "optimal_slack"() -> (w859:string)
            n326 = call "PID2_2V.vi"("V_afe"=w824, "V_up"=w825) -> ()  [unwired: 9 in, 1 out]
            n327 = call "distribute_setpoints_DC.vi"("setpoints"=w844) -> ("reference_DC"=w837:T17)  [unwired: 10 in]
            n328 = Bundle(cluster=T35 {"Frequency"=0.0, "Angle"=0.0, "Magnitude"=0.0} ("upper layer grid info"), "Frequency"=50.0, "Angle"=0.0, "Magnitude"=w821) -> (w840:T35)
            n329 = local read "SC_soc"() -> (w834:dbl)
            n330 = local read "SC_soc"() -> (w835:dbl)
            n331 = call "distribute_setpoints.vi"("setpoints"=w848, "upper layer grid info"=w840) -> ("references"=w849:T21)  [unwired: 9 in]
            n332 = local write "V_upstream"(w825) -> ()
            n333 = local write "V_afe"(w824) -> ()
            n334 = Bundle("V_control_fix_for_island"=w821) -> (w823:cluster{"V_control_fix_for_island":dbl})  [unwired: 1 in]
            n335 = Bundle By Name(cluster=w852, "Data.Operation_mode"="Island" ("Operation_mode"), "Data.Optimal_slack"=w859, "Data.upper_layer_grid_info"=w827, "Data.SC_soc"=w835, "Data.P_pv_facade"=w828, "Data.PV"=w832) -> (w855:T1)
            n336 = Bundle By Name(cluster=w833, "Data.Operation_mode"="Island" ("Operation_mode"), "Data.Optimal_slack"=w860, "Data.upper_layer_grid_info"=w827, "Data.SC_soc"=w834, "Data.P_pv_facade"=w828, "Data.PV"=w832) -> (w856:T1)
            n337 = Bundle By Name(cluster=w847, "Data.Start following"=FALSE, "Data.Start forming"=TRUE, "Data.SC references"=w837) -> (w846:T12)
            n338 = Bundle By Name(cluster=w850, "Data.close/open relay"=FALSE, "Data.Operation mode"="Island" ("Operation_mode")) -> (w853:T22)
            n339 = local write "V control"(w823) -> ()
            n340 = Bundle By Name(cluster=w851, "Data.Start forming 2"=FALSE, "Data.Start following 2"=TRUE, "Data.Start following 1"=FALSE, "Data.Start forming 1"=TRUE, "Data.references"=w849) -> (w854:T18)
            n341 = local write "Reset_magnitude"(FALSE ("Rest_PI_V")) -> ()
          }
        }
        n342 = case shown="True" "to prepare for grid connection" {
          tunnel: [State_Machine."Island" ("State") State_Machine."Prepare for connection" ("State")] -> w758
          tunnel: w750 -> [w780 w783]
          tunnel: [w780 w783] -> w749
          frame False {
          }
          frame True {
            # "only go to next state if OPFs are feasible\n for 7 timesteps"
            n343 = local write "Reset_angle"(TRUE ("Reset_angle")) -> ()
            n344 = local write "delta angle"(0.0 ("delta angle")) -> ()
            n345 = local write "Reset_magnitude"(TRUE ("Rest_PI_V")) -> ()
          }
        }
      }
      frame "Prepare for connection" {
        # "prepare for connection - Display a dialog box with a message specific to State 3, then go back to the Wait for Event state."
        n346 = flat-sequence {
          tunnel: w900 -> [w932]
          tunnel: w899 -> [w933]
          tunnel: w898 -> [w934]
          tunnel: w897 -> [w935]
          tunnel: [w935] -> w890
          tunnel: [w934] -> w889
          tunnel: [w933] -> w888
          tunnel: [w932] -> w887
          tunnel: [w908] -> w886
          tunnel: [w913] -> w885
          tunnel: w884 -> [w926]
          tunnel: [w926] -> w883
          tunnel: [w908] -> w882
          tunnel: [w923] -> w878
          tunnel: [w918] -> w877
          tunnel: [w919] -> w876
          tunnel: w875 -> [w921]
          tunnel: [w920] -> w874
          tunnel: w871 -> [w916]
          tunnel: [w915] -> w870
          tunnel: [w911] -> w869
          tunnel: [w914] -> w868
          tunnel: [w910] -> w867
          tunnel: w866 -> [w910]
          tunnel: ["Reset_angle"] -> w863
          tunnel: [w908] -> w861
          tunnel: w890 -> [w984]
          tunnel: w889 -> [w983]
          tunnel: w888 -> [w982]
          tunnel: w887 -> [w981]
          tunnel: w886 -> [w979]
          tunnel: w885 -> [w968]
          tunnel: w883 -> [w978]
          tunnel: w882 -> [w974]
          tunnel: [w988] -> w894
          tunnel: [w987] -> w893
          tunnel: [w986] -> w892
          tunnel: [w985] -> w891
          tunnel: [w977] -> w881
          tunnel: w878 -> [_]
          tunnel: w877 -> [w963]
          tunnel: w876 -> [w962]
          tunnel: w874 -> [w959]
          tunnel: w870 -> [w953]
          tunnel: w869 -> [w952]
          tunnel: w868 -> [w954]
          tunnel: [w949] -> w865
          tunnel: w867 -> [w949]
          tunnel: w863 -> [w947]
          tunnel: [w943] -> w862
          tunnel: w861 -> [w943]
          frame #0 {
            # "from island OPF"
            # "from connected OPF"
            # "from resource"
            # "from synchrocheck"
            n347 = Unbundle By Name(w916) -> ("Data.Voltage mag"=w917:dbl[])  [unwired: 1 out]
            n348 = Unbundle By Name(w921) -> ("Data.PV_mpp"=w920:T36)
            n349 = Unbundle By Name(w926) -> ("Data.Forming/Following"=w927:bool, "Data.measurements SC.SOC"=w922:dbl)
            n350 = Unbundle By Name(w935) -> ("Data.solution_feasible"=w931:dbl, "Data.setpoints"=w908:dbl[], "Data.upper_layer_grid_info"=w923:T35)
            n351 = Unbundle By Name(w933) -> ("Data.Forming/Following"=w942:bool[])
            n352 = Unbundle By Name(w932) -> ("Data.Synchronised?"=w937:bool, "Data.V_UpStream"=w925:T25, "Data.V_Downstream"=w924:T25)
            n353 = Unbundle By Name(w934) -> ("Data.solution_feasible"=w929:dbl)  [unwired: 1 out]
            n354 = local write "to grid connection"(FALSE ("to grid connection")) -> ()
            n355 = local write "to prepare for island"(FALSE ("to prepare for island")) -> ()
            n356 = local write "to island"(FALSE ("to island")) -> ()
            n357 = local write "to prepare for grid connection"(TRUE ("to prepare for grid connection")) -> ()
            n358 = Index Array(array=w917, index=0) -> (element=w911:dbl)
            n359 = Not Equal To 0?(x=w929) -> (x != 0?=w928:bool)
            n360 = Not Equal To 0?(x=w931) -> (x != 0?=w930:bool)
            n361 = local write "synchronised?"(w937) -> ()
            n362 = local read "Reset_magnitude"() -> (w914:bool)
            n363 = Or Array Elements(Boolean array=w942) -> (logical OR=w936:bool)
            n364 = local write "forming SC?"(w927) -> ()
            n365 = local write "setpoints"(w908) -> ()
            n366 = local write "SC_soc"(w922) -> ()
            n367 = local write "cOPF valid?"(w928) -> ()
            n368 = local write "iOPF valid"(w930) -> ()
            n369 = local write "forming AFE?"(w936) -> ()
            n370 = call "up_grid_data_prepareConnection.vi"("Data.V_Downstream"=w924, "Data.V_UpStream"=w925) -> ("upper layer grid info"=w913:T35, "DOWN_Angle_unwrap"=w919:dbl, "UP_Angle_unwrap"=w918:dbl)  [unwired: 5 in, 2 out]
            n371 = Unbundle By Name(w913) -> ("Magnitude"=w915:dbl)
          }
          frame #1 {
            # "reduce K_p, so we don't have a step"
            # "send to island OPF"
            # "send to connected OPF"
            # "send to resource"
            # "send to synchrocheck"
            n372 = Subtract(x=w963, y=w962) -> (x-y=w945:dbl)
            "delta angle" <- w945
            n373 = Unbundle(w968) -> ()  [unwired: 3 out]
            n374 = call "PID2.vi"("Rest_PI_theta"=w947, "input"=w962, "setpoint"=w963) -> ("output"=w965:dbl)  [unwired: 8 in]
            n375 = call <userlib>:"Boolean Trigger__ogtk.vi"("Boolean Input"=w954) -> ("Rising Edge"=w955:bool)  [unwired: 1 in, 1 out]
            n376 = local read "P_pv_facade"() -> (w956:dbl)
            n377 = local read "optimal_slack"() -> (w991:string)
            n378 = local read "optimal_slack"() -> (w992:string)
            n379 = call "PID2_2V.vi"("reinitialize? (F)"=w955, "V_afe"=w952, "V_up"=w953) -> ("output"=w948:dbl)  [unwired: 8 in]
            n380 = local read "SC_soc"() -> (w960:dbl)
            n381 = Bundle(cluster=T35 {"Frequency"=0.0, "Angle"=0.0, "Magnitude"=0.0} ("upper layer grid info"), "Frequency"=w965, "Angle"=0.0, "Magnitude"=w948) -> (w969:T35)
            n382 = local read "SC_soc"() -> (w961:dbl)
            n383 = call "distribute_setpoints_DC.vi"("setpoints"=w974) -> ("reference_DC"=w975:T17)  [unwired: 10 in]
            n384 = Bundle(w945) -> (→"V angle":cluster{dbl})  [unwired: 1 in]
            n385 = call "distribute_setpoints.vi"("setpoints"=w979, "upper layer grid info"=w969) -> ("references"=w980:T21)  [unwired: 9 in]
            n386 = local write "V_upstream"(w953) -> ()
            n387 = local write "V_afe"(w952) -> ()
            n388 = Bundle By Name(cluster=w983, "Data.Operation_mode"="Prepare for connection" ("Operation_mode"), "Data.Optimal_slack"=w991, "Data.upper_layer_grid_info"=w968, "Data.SC_soc"=w960, "Data.P_pv_facade"=w956, "Data.PV"=w959) -> (w987:T1)
            n389 = Bundle By Name(cluster=w984, "Data.Operation_mode"="Prepare for connection" ("Operation_mode"), "Data.Optimal_slack"=w992, "Data.upper_layer_grid_info"=w968, "Data.SC_soc"=w961, "Data.P_pv_facade"=w956, "Data.PV"=w959) -> (w988:T1)
            n390 = Bundle("output"=w948) -> (w951:cluster{"output":dbl})  [unwired: 1 in]
            n391 = Bundle By Name(cluster=w978, "Data.Start following"=FALSE, "Data.Start forming"=TRUE, "Data.SC references"=w975) -> (w977:T12)
            n392 = Bundle By Name(cluster=w981, "Data.close/open relay"=FALSE, "Data.Operation mode"="Prepare for connection" ("Operation_mode")) -> (w985:T22)
            n393 = local write "V_control"(w948) -> ()
            n394 = Bundle By Name(cluster=w982, "Data.Start forming 2"=FALSE, "Data.Start following 2"=TRUE, "Data.Start following 1"=FALSE, "Data.Start forming 1"=TRUE, "Data.references"=w980) -> (w986:T18)
            n395 = local write "Reset_angle"(FALSE ("Reset_angle")) -> ()
            n396 = local write "Reset_magnitude"(FALSE ("Rest_PI_V")) -> ()
            n397 = local write "V control"(w951) -> ()
          }
        }
        n398 = local read "synchronised?"() -> (w872:bool)
        n399 = And(x="to grid connection", y=w872) -> (x .and. y?=w873:bool)
        n400 = case shown="True" w873 {
          tunnel: [State_Machine."Prepare for connection" ("State") State_Machine."Grid connected" ("State")] -> w879
          tunnel: w865 -> [w901 w905]
          tunnel: [w901 w905] -> w864
          tunnel: w862 -> [_ w904]
          frame False {
          }
          frame True {
            # "only go to next state if OPFs are feasible\n for 7 timesteps"
            n401 = local write "Reset_magnitude"(TRUE ("Rest_PI_V")) -> ()
            "old_sp_island" <- w904
            "old_sp_island_bool" <- TRUE ("Data.Start forming 1")
          }
        }
      }
    }
    "OUT Synchro" <- w415
    "OUT AFE" <- w414
    "OUT cOPF" <- w413
    "OUT iOPF" <- w412
    "OUT PV+SC" <- w403
    n402 = node-c288() -> ()  [unwired: 1 in, 1 out]
  }
  n403 = call-poly <vilib>:"Read Delimited Spreadsheet.vi"("file path (dialog if empty)"=path "C:/Users/admin/Documents/git-clones/acdc_centralized_controller2/Data/Zenone_profile.csv", "format (%.3f)"="%.3f", "delimiter (\\t)"=" " ("delimiter (\\t)")) -> ("all rows"=w37:dbl[][])  [unwired: 7 in, 5 out]
  n404 = node-c288(w5) -> ()  [unwired: 1 out]
  n405 = UDP Close(connection ID=w90, 8:w89) -> ()  [unwired: 2 out]
  n406 = UDP Close(connection ID=w14, 8:w13) -> ()  [unwired: 2 out]
  n407 = UDP Close(connection ID=w25, 8:w26) -> ()  [unwired: 2 out]
  n408 = Matrix Size(0:w37) -> (1:w24:i32)  [unwired: 1 out]
  n409 = UDP Close(connection ID=w33, 8:w48) -> ()  [unwired: 2 out]
  n410 = while {
    shift-right: [w1005] -> _
    shift-left: 0 ("number of rows") -> [w1003]
    tunnel: w37 -> [w998]
    tunnel: w24 -> [w999]
    stop <- w1006 stop-if-true
    (unwired) 3.0 ("element")
    (unwired) 6.0 ("element")
    n411 = Quotient & Remainder(x=w1003, y=w999) -> (x-y*floor(x/y)=w1002:i32)  [unwired: 1 out]
    n412 = Index Array(array=w998, index (row)=w1002) -> (element=w996:dbl[])  [unwired: 1 in]
    n413 = Multiply(x=0.66 ("Numeric"), y=w996) -> (x*y=w997:dbl[])
    n414 = Index Array(array=w997) -> (element #1=w994:dbl, element #2=w993:dbl)  [unwired: 2 in]
    n415 = Absolute Value(x=w993) -> (abs(x)=→"Zenone_Q":dbl)
    n416 = Absolute Value(x=w994) -> (abs(x)=→"Zenone_P":dbl)
    n417 = local read "Stop"() -> (w1006:bool)
    n418 = Increment(x=w1002) -> (x+1=w1005:i32)
    n419 = Wait (ms)(milliseconds to wait=u32 1000) -> ()  [unwired: 1 out]
  }
  n420 = node-c288(w8) -> ()  [unwired: 1 out]
  n421 = UDP Close(connection ID=w54, 8:w53) -> ()  [unwired: 2 out]
  n422 = UDP Close(connection ID=w92, 8:w91) -> ()  [unwired: 2 out]
  n423 = UDP Close(connection ID=w58, 8:w57) -> ()  [unwired: 2 out]
  n424 = UDP Close(connection ID=w56, 8:w55) -> ()  [unwired: 2 out]
  n425 = node-c288(w106) -> ()  [unwired: 1 out]
